vi "script_processor.vi"(7 "Ref_RunScriptWindow":refnum<vi>, 8 "error in (no error)":errorcluster, 10 "command":string) -> (0 "error out":errorcluster)   [LabVIEW 2017]
doc: "This is the main VI that processes all the script command. Here are all the functions listed and processed"
uses:
  Classes/Flags/flag.lvclass
  Classes/Plots/Plots.lvclass
  global variables.vi
  Classes/StatusLog/StatusLog.lvclass
  Classes/Message/Message.lvclass
  Classes/PrepLineObject/PrepLineObject.lvclass
  Classes/Standard/Standard.lvclass
  Classes/Pipette/Pipette.lvclass
  Classes/Instrument/instrument.lvclass
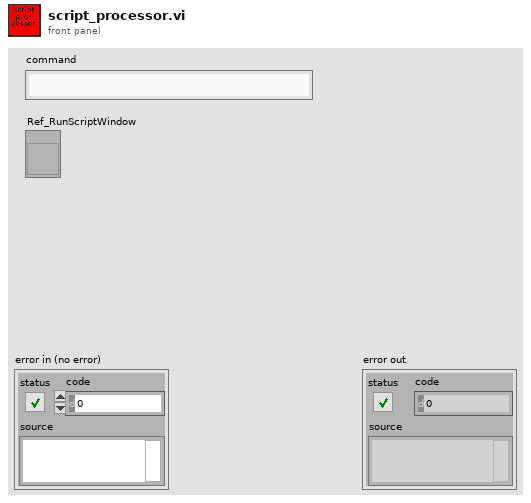
[diagram p1: front panel]
types:
  T1 = cluster{"plot command":string, "Variant":variant}
  T2 = cluster{"format string":string, "Variant":variant}
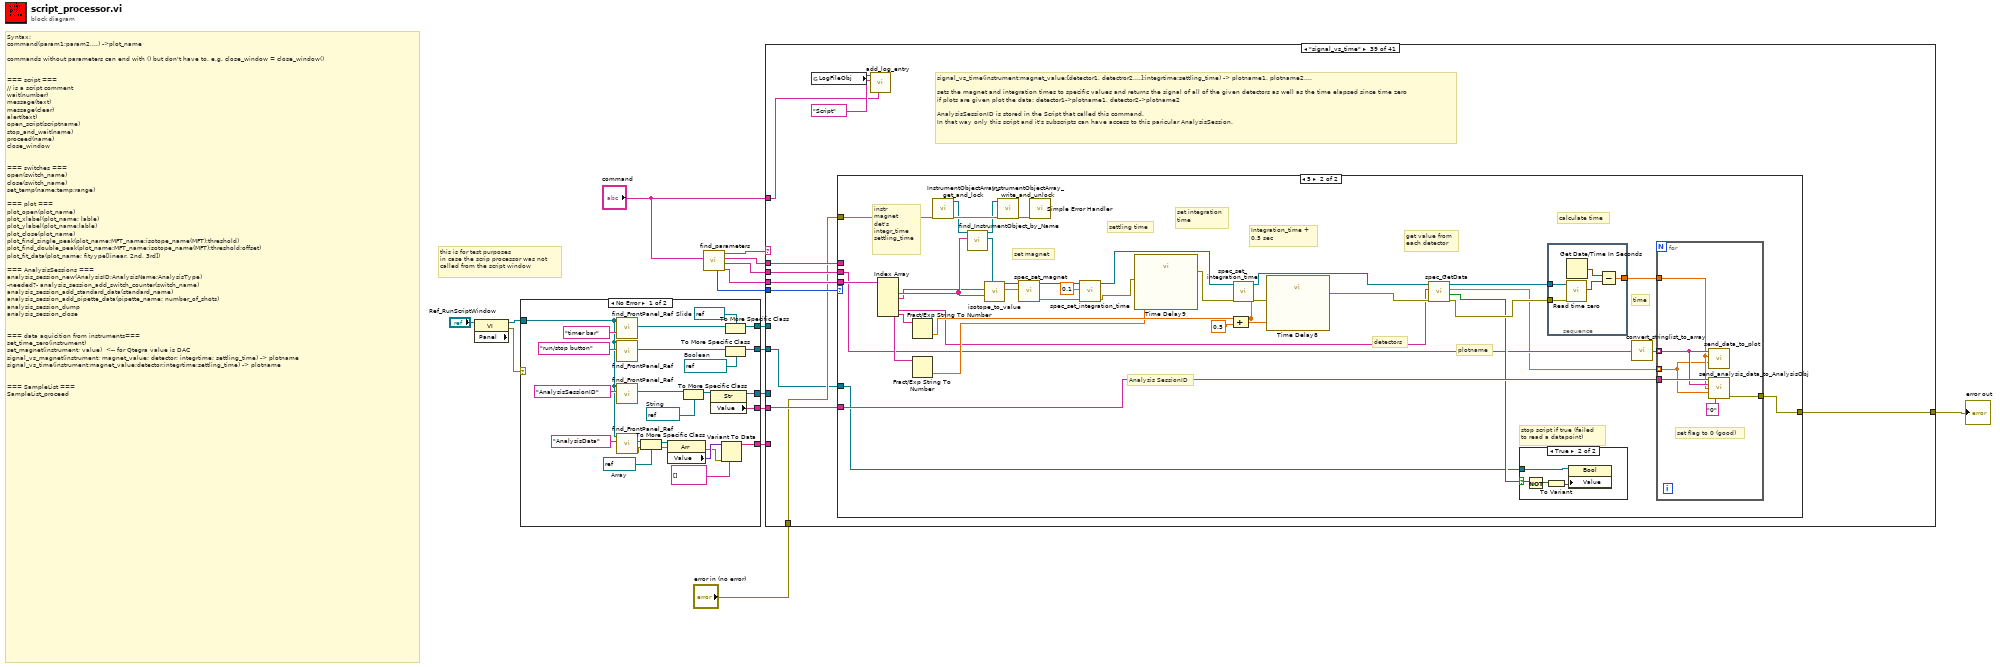
[diagram p0: block diagram]
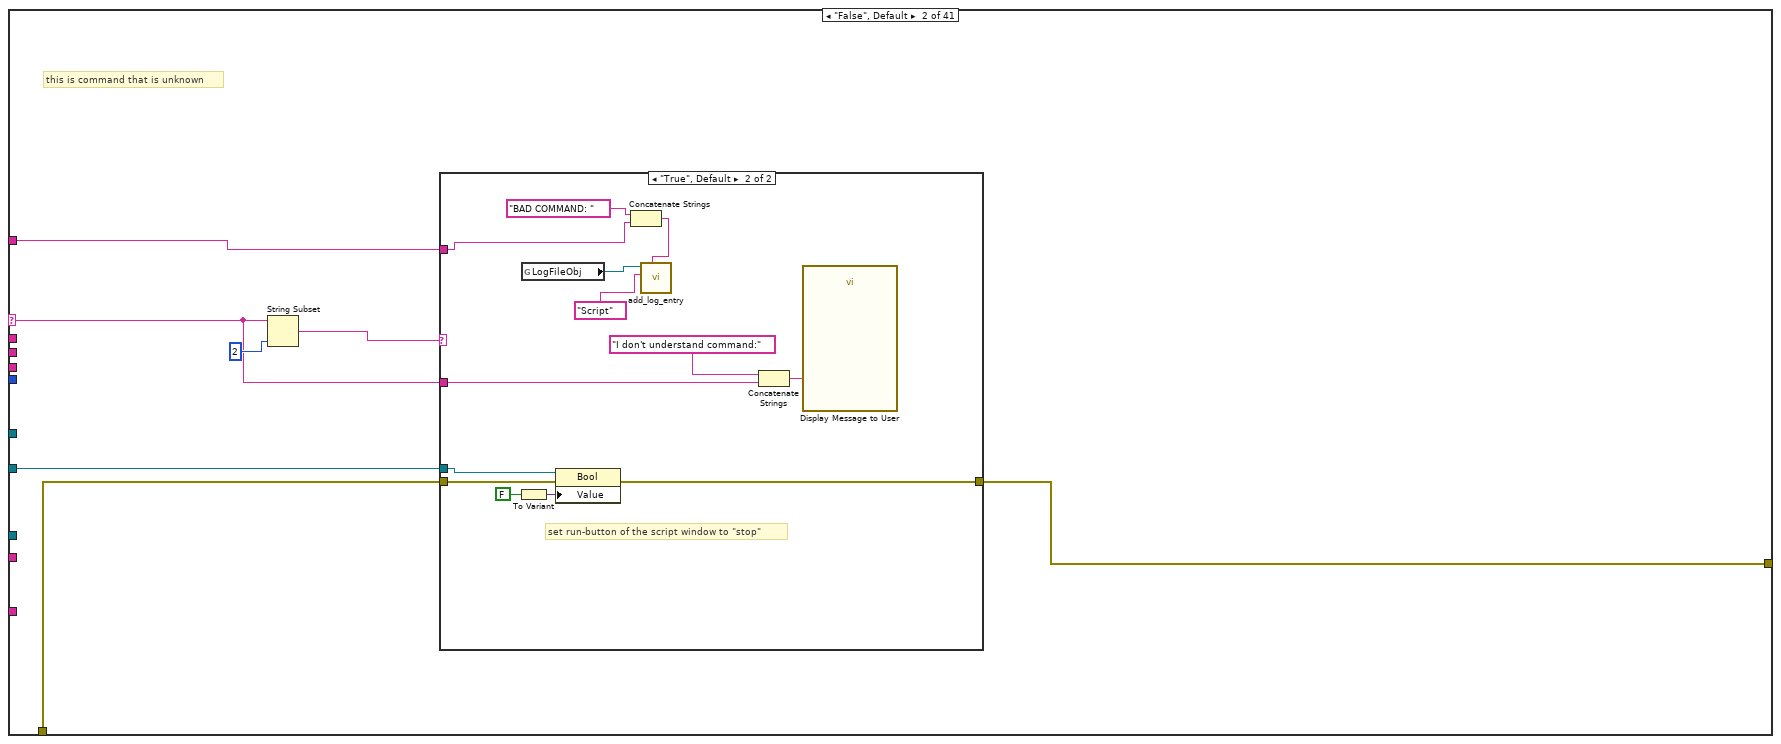
[diagram p4: hidden frame]
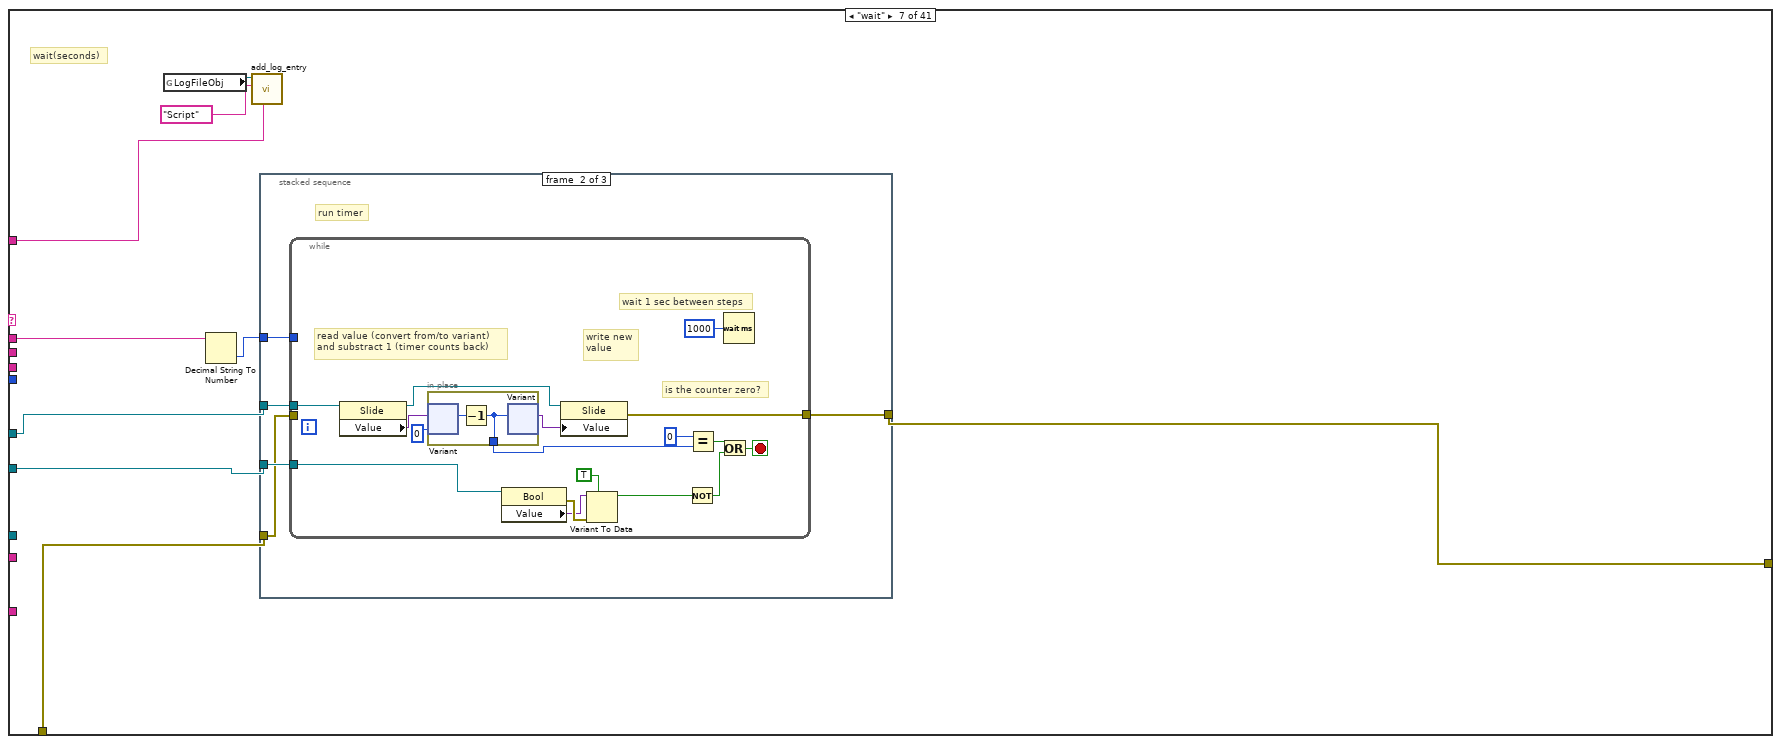
[diagram p10: hidden frame]
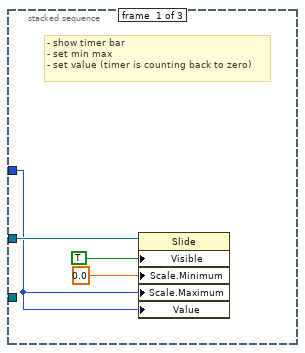
[diagram p11: hidden frame]
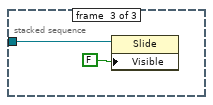
[diagram p12: hidden frame]
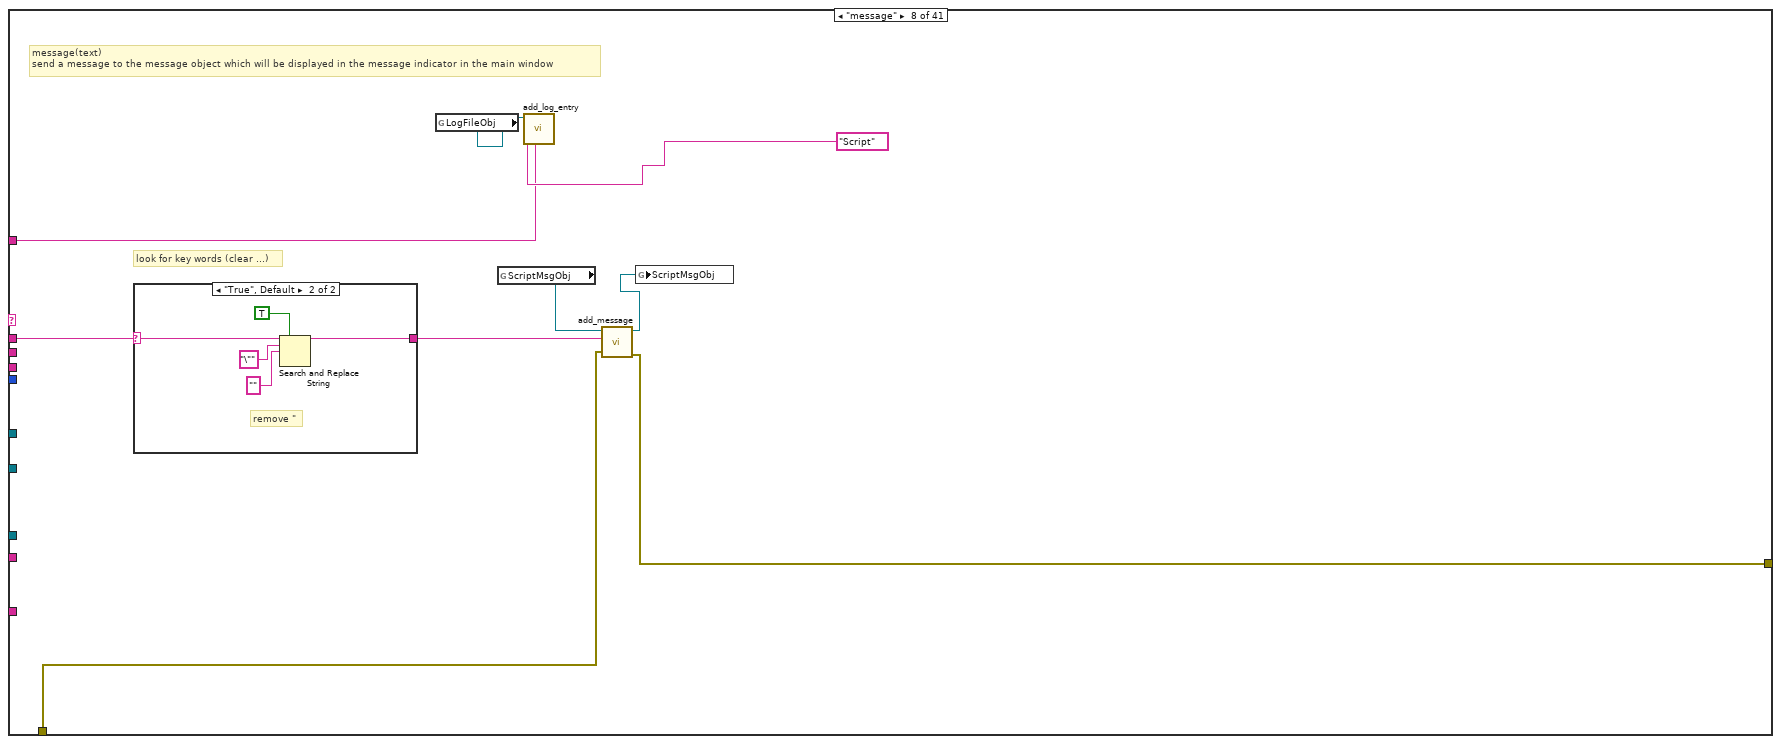
[diagram p13: hidden frame]
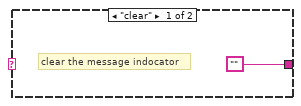
[diagram p14: hidden frame]
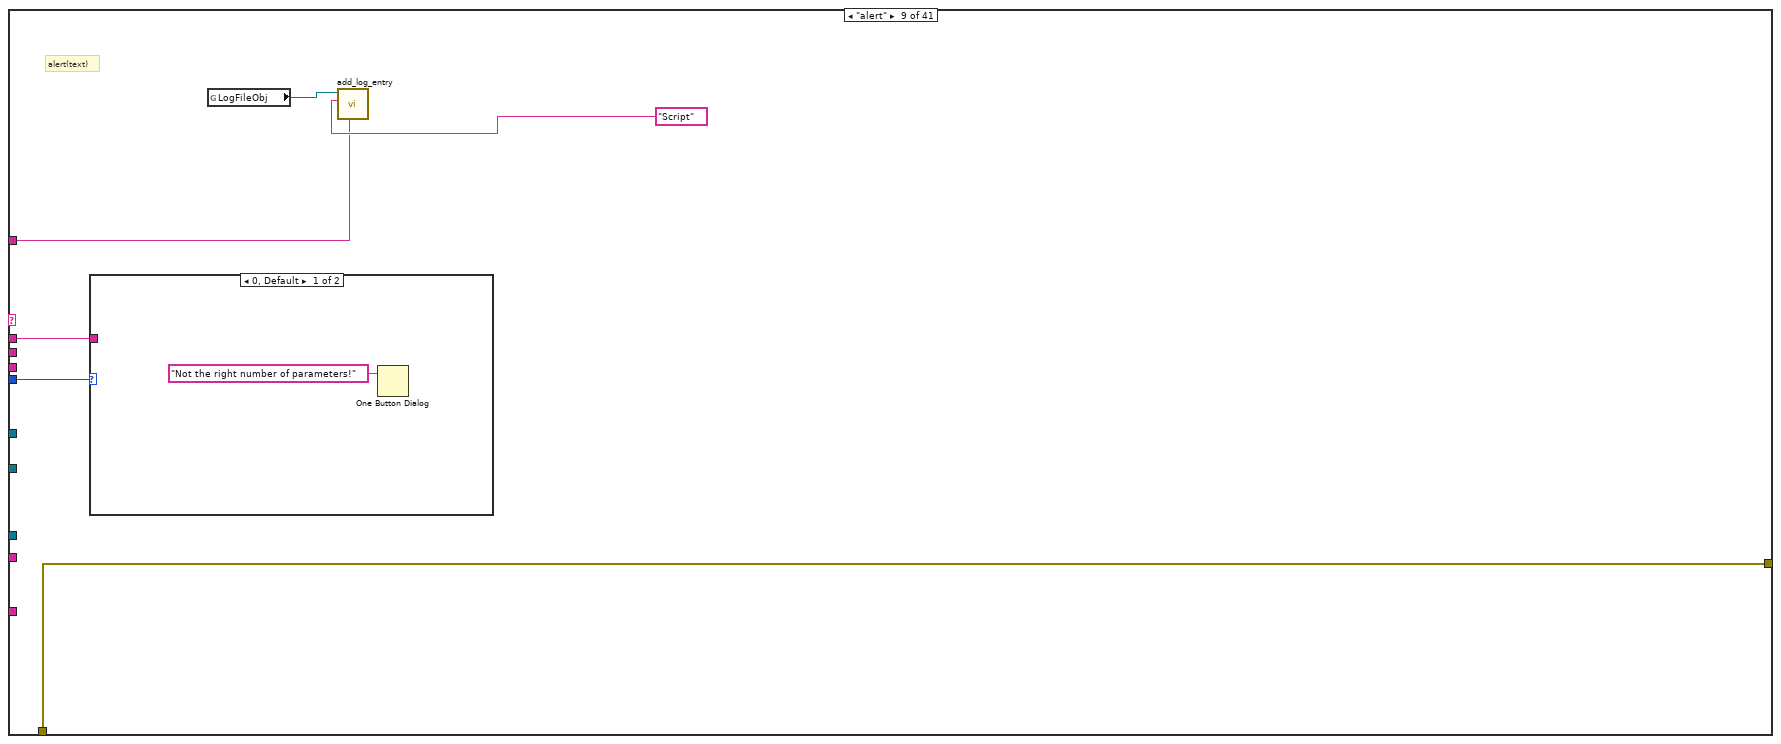
[diagram p15: hidden frame]
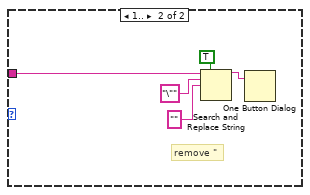
[diagram p16: hidden frame]
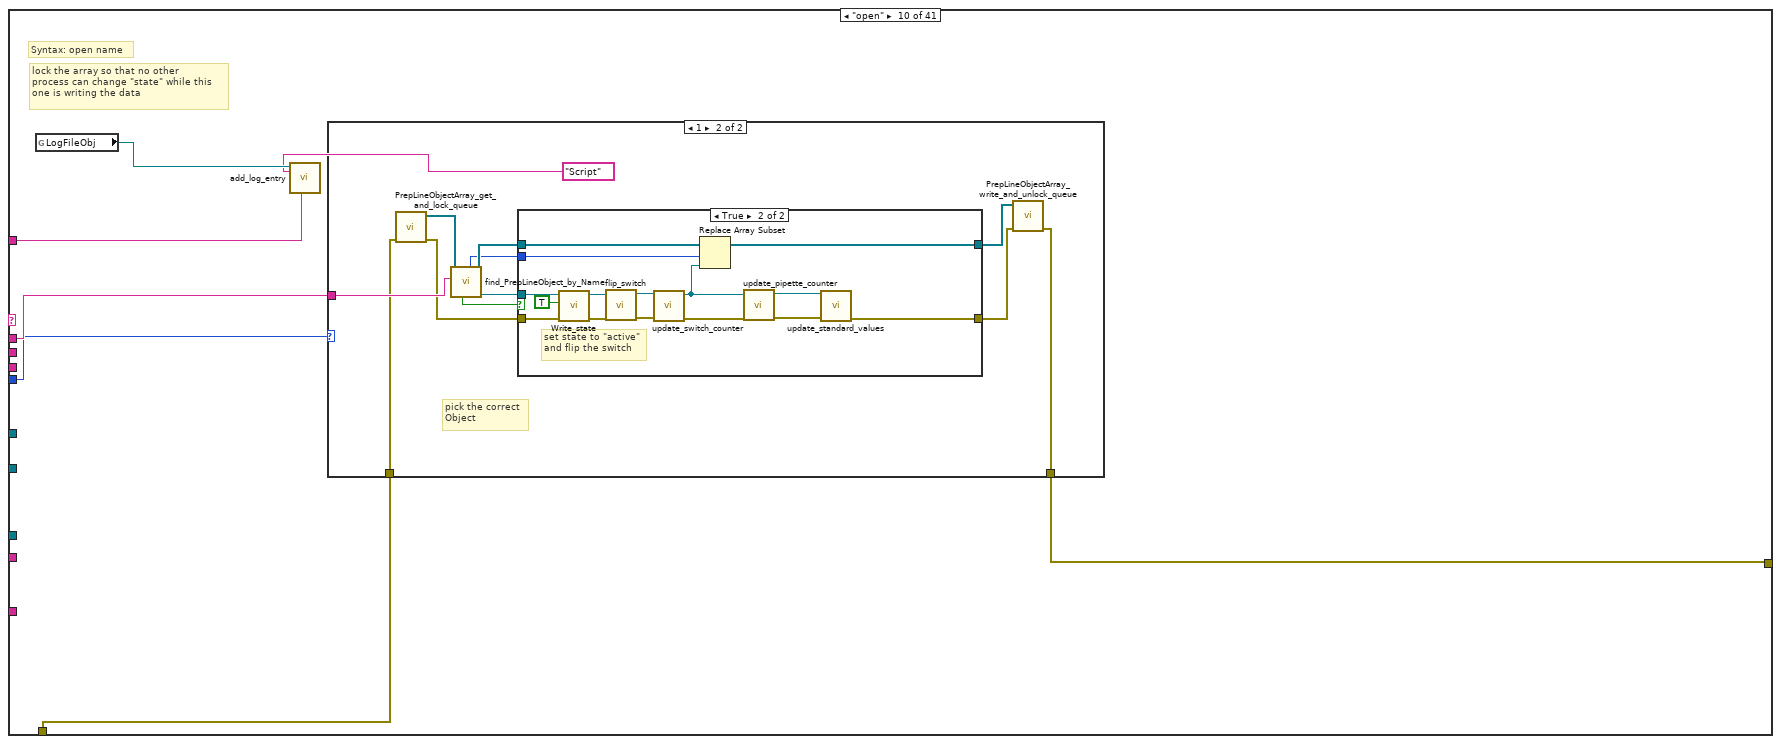
[diagram p17: hidden frame]
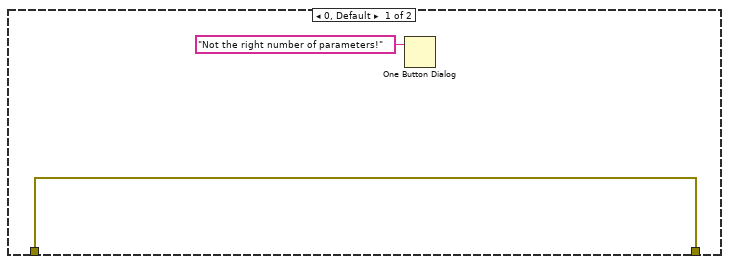
[diagram p18: hidden frame]
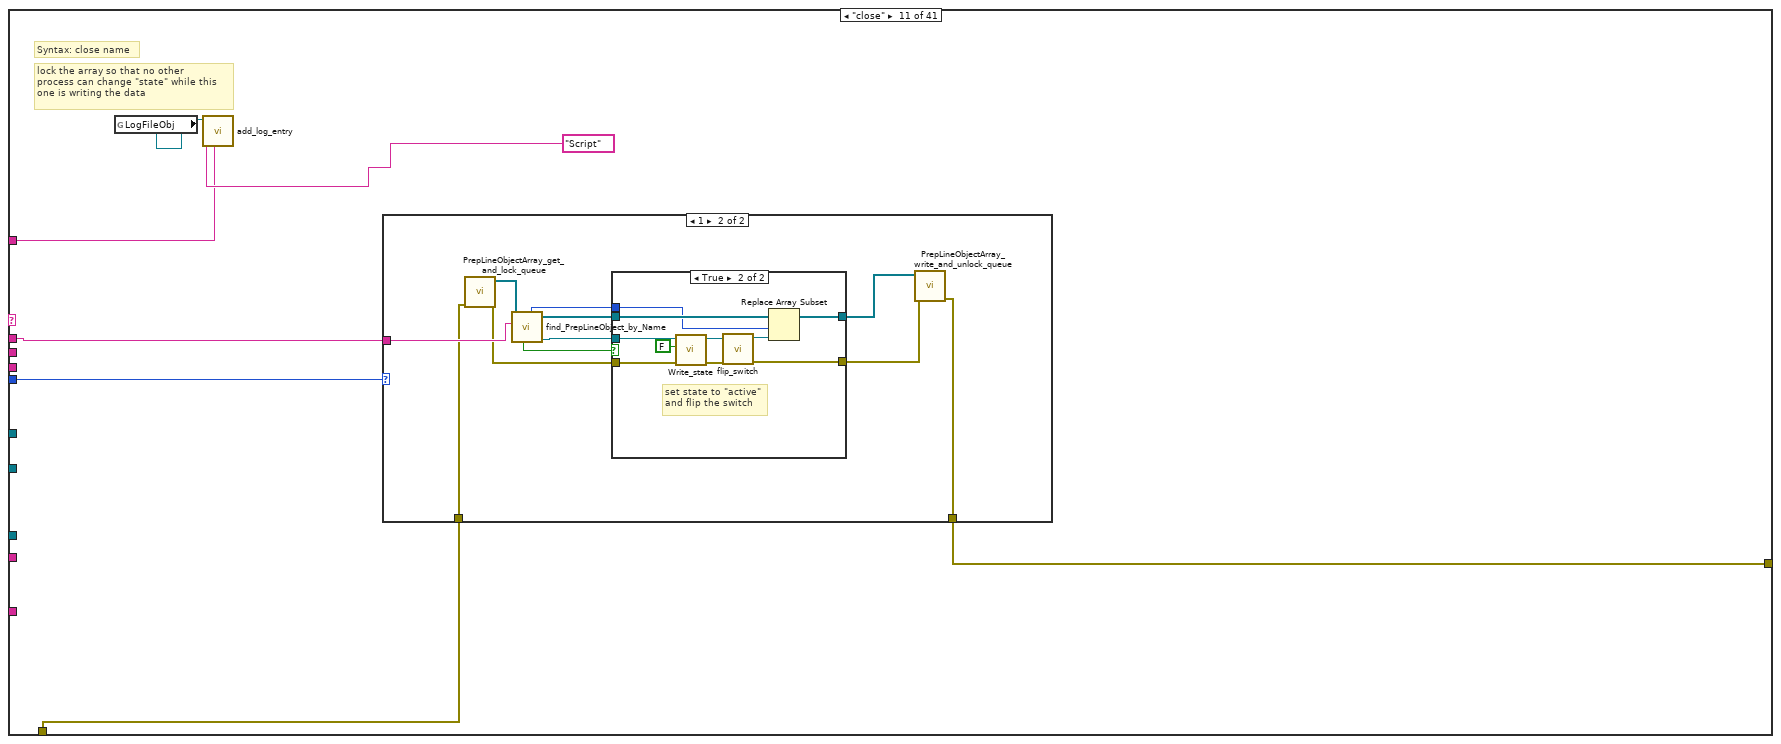
[diagram p20: hidden frame]
diagram:
  # "this is for test purposes\nin case the scrip processor was not\ncalled from the script window"
  # "Syntax:\ncommand(param1;param2,...) ->plot_name\n\ncommands without parameters can end with () but don't have to, e.g. close_window = close_window()\n\n\n=== script ===\n// is a script comment\nwait(number)\nmessage(text)\nmessage(clear)\nalert(text)\nopen_script(scriptname)\nstop_and_wait(name)\nproceed(name)\nclose_window\n\n\n=== switches ===\nopen(switch_name)\nclose(switch_name)\nset_temp(name;temp;range)\n\n=== plot ===\nplot_open(plot_name)\nplot_xlabel(plot_name; lable)\nplot_ylabel(plot_name;lable)\nplot_close(plot_name)\nplot_find_single_peak(plot_name;MFT_name;isotope_name(MFT);threshold)\nplot_find_double_peak(plot_name;MFT_name;isotope_name(MFT);threshold;offset)\nplot_fit_data(plot_name; fityype[linear, 2nd, 3rd])\n\n=== AnalysisSessions ===\nanalysis_session_new(AnalysisID;AnalysisName;AnalysisType)\n-needed?- analysis_session_add_switch_counter(switch_name)\nanalysis_session_add_standard_data(standard_name)\nanalysis_session_add_pipette_data(pipette_name; number_of_shots)\nanalysis_session_dump\nanalysis_session_close\n\n\n=== data aquicition from instruments===\nset_time_zero(instrument)\nset_magnet(instrument; value)  <-- for Qtegra value is DAC\nsignal_vs_magnet(instrument; magnet_value; detector; integrtime; settling_time) -> plotname\nsignal_vs_time(instrument;magnet_value;detector;integrtime;settling_time) -> plotname\n\n\n=== SampleList ===\nSampleList_proceed"
  n1 = property class="VI" props=["Panel"](reference="Ref_RunScriptWindow") -> (reference out=w5:refnum<vi>, error out=w4:errorcluster)  [unwired: 1 in, 1 out]
  n2 = case shown="No Error" w4 {
    tunnel: [w36 _] -> w14
    tunnel: [w35 _] -> w13
    tunnel: w5 -> [w17 _]
    tunnel: [w29 _] -> w3
    tunnel: [w28 _] -> w2
    tunnel: [w22 _] -> w1
    frame No Error {
      w25 = refnum<vi> refnum  # Array
      w32 = refnum<vi> refnum  # String
      w34 = refnum<vi> refnum  # Boolean
      w37 = refnum<vi> refnum  # Slide
      n3 = call "find_FrontPanel_Ref.vi"("FrontPanelObject name"="timer bar", "Ref_RunScriptWindow"=w17) -> ("FrontPanelObject ref out"=w39:refnum<vi>)  [unwired: 7 in, 2 out]
      n4 = call "find_FrontPanel_Ref.vi"("FrontPanelObject name"="run/stop button", "Ref_RunScriptWindow"=w17) -> ("FrontPanelObject ref out"=w38:refnum<vi>)  [unwired: 7 in, 2 out]
      n5 = call "find_FrontPanel_Ref.vi"("FrontPanelObject name"="AnalysisSessionID", "Ref_RunScriptWindow"=w17) -> ("FrontPanelObject ref out"=w31:refnum<vi>)  [unwired: 7 in, 2 out]
      n6 = call "find_FrontPanel_Ref.vi"("FrontPanelObject name"="AnalysisData", "Ref_RunScriptWindow"=w17) -> ("error out"=w20:errorcluster, "FrontPanelObject ref out"=w26:refnum<vi>)  [unwired: 7 in, 1 out]
      n7 = To More Specific Class(target class=w25, reference=w26, error in=w20) -> (specific class reference=w27:refnum<vi>, error out=w19:errorcluster)
      n8 = property class="Arr"(reference=w27, error in=w19) -> (error out=w18:errorcluster, "Value"=w21:variant)  [unwired: 1 out]
      n9 = To More Specific Class(target class=w32, reference=w31) -> (specific class reference=w30:refnum<vi>)  [unwired: 1 in, 1 out]
      n10 = property class="Str"(reference=w30) -> (reference out=w28:refnum<vi>, "Value"=w29:string)  [unwired: 1 in, 1 out]
      n11 = Variant To Data(error in=w18, type=string[] [], Variant=w21) -> (data=w22:string[])  [unwired: 1 out]
      n12 = To More Specific Class(target class=w37, reference=w39) -> (specific class reference=w36:refnum<vi>)  [unwired: 1 in, 1 out]
      n13 = To More Specific Class(target class=w34, reference=w38) -> (specific class reference=w35:refnum<vi>)  [unwired: 1 in, 1 out]
    }
    frame Error {
    }
  }
  n14 = call "find_parameters.vi"("script input"="command") -> ("Parameter Array"=w8:string[], "plotnames (string list)"=w9:string, "parameter string"=w10:string, "command"=w11:string, "number of parameters"=w7:u8)  [unwired: 6 in]
  n15 = case shown="\"signal_vs_time\"" w11 {
    selector: w11 -> [_ w47 _ _ _ _ _ _ _ _ _ _ _ _ _ _ _ _ _ _ _ _ _ _ _ _ _ _ _ _ _ _ _ _ _ _ _ _ _ _ _]
    tunnel: w10 -> [_ _ _ _ _ _ w76 w110 w127 w140 w177 w211 w270 w298 w353 _ w403 w437 w453 w463 w498 w557 w623 _ _ w718 w747 w776 _ w820 w857 w886 w917 w948 w989 w1022 w1053 w1103 w1164 w1227 _]
    tunnel: w13 -> [_ w46 _ _ _ _ w73 _ _ _ _ w210 w261 w297 _ _ _ _ _ _ _ _ _ _ _ _ _ _ _ _ _ _ _ _ _ _ w1046 w1096 w1157 _ _]
    tunnel: "error in (no error)" -> [w42 w45 w64 w65 w66 w67 w72 w113 w122 w139 w176 w209 w269 w291 w352 w390 w410 w436 w452 w468 w499 w558 w624 w683 w712 w715 w744 w773 _ w819 w853 w882 w913 w944 w985 w1018 w1047 w1097 w1158 w1224 w1261]
    tunnel: [w42 w44 w64 w65 w66 w67 w71 w112 w122 w138 w175 w208 w268 w296 w351 w389 w409 w435 w451 w467 w497 w556 w622 w682 w711 w719 w748 w777 _ w818 w852 w881 w912 w943 w984 w1017 w1052 w1101 w1162 _ w1260] -> w15
    tunnel: "command" -> [_ w43 _ _ _ _ w68 w107 w124 w135 w172 w205 w265 w293 w349 w386 w406 w432 w448 w464 w500 w559 w625 w686 w707 w720 w749 w778 w806 w821 w855 w884 w915 w946 w987 w1020 w1054 w1104 w1165 w1229 w1257]
    tunnel: w14 -> [_ _ _ _ _ _ w74 _ _ _ _ _ _ _ _ _ _ _ _ _ _ _ _ _ _ _ _ _ _ _ _ _ _ _ _ _ _ _ _ _ _]
    tunnel: w9 -> [_ _ _ _ _ _ _ _ _ _ _ _ _ _ _ _ _ _ _ _ _ _ _ _ _ _ _ _ _ _ _ _ _ _ _ _ w1051 w1102 w1163 w1226 _]
    tunnel: w8 -> [_ _ _ _ _ _ _ _ _ _ _ w203 _ _ _ _ w404 w430 w446 _ w495 w554 w620 w677 _ _ _ _ _ _ w851 w880 w911 w942 w983 w1016 w1049 w1099 w1160 w1225 _]
    tunnel: w7 -> [_ _ _ _ _ _ _ _ w123 w134 w171 w204 w264 w292 w348 _ w405 w431 w447 w462 w496 w555 w621 _ _ w717 w746 w775 _ w817 w854 w883 w914 w945 w986 w1019 w1050 w1100 w1161 w1228 _]
    tunnel: w3 -> [_ _ _ _ _ _ _ _ _ _ _ _ w263 _ _ _ _ _ _ _ w494 w553 w619 _ w705 w716 w745 w774 w809 _ _ _ _ _ _ _ w1048 w1098 w1159 w1223 _]
    tunnel: w2 -> [_ _ _ _ _ _ _ _ _ _ _ _ _ _ _ _ _ _ _ _ _ _ _ w679 _ _ _ _ _ _ _ _ _ _ _ _ _ _ _ _ _]
    tunnel: w1 -> [_ _ _ _ _ _ _ _ _ _ _ _ _ _ _ _ _ _ _ _ _ _ _ w675 _ _ _ _ _ _ _ _ _ _ _ _ _ _ _ _ _]
    frame "" {
      # "empty line"
    }
    frame "False", Default {
      # "this is command that is unknown"
      n16 = String Subset(string=w47, length (rest)=2 ("length (rest)")) -> (substring=w48:string)  [unwired: 1 in]
      n17 = case shown="\"True\", Default" w48 {
        tunnel: w47 -> [_ w61]
        tunnel: w46 -> [_ w57]
        tunnel: w45 -> [w50 w58]
        tunnel: [w50 w56] -> w44
        tunnel: w43 -> [_ w51]
        frame "//" {
          # "this is a comment that has no space after it"
        }
        frame "True", Default {
          # "set run-button of the script window to \"stop\""
          n18 = To Variant(anything=FALSE) -> (Variant=w60:variant)
          n19 = global read "global variables.vi" "LogFileObj"() -> (w52:refnum<class "StatusLog.lvclass">)
          n20 = property class="Bool"(reference=w57, error in=w58, "Value"=w60) -> (error out=w56:errorcluster)  [unwired: 1 out]
          n21 = Concatenate Strings("BAD COMMAND: ", w51) -> (w55:string)
          n22 = call-dynamic "add_log_entry.vi"("new entry"=w55, "log identifiers"="Script", "StatusLog in"=w52) -> ()  [unwired: 5 in, 2 out]
          n23 = Concatenate Strings("I don't understand command:" ("Message"), w61) -> (w62:string)
          n24 = call "Display Message to User"("Message"=w62) -> ()  [unwired: 9 in, 2 out]
        }
      }
    }
    frame "\n" {
      # "empty line"
    }
    frame "\r" {
    }
    frame "\n\r" {
    }
    frame "//" {
      # "this is a script comment"
    }
    frame "wait" {
      # "wait(seconds)"
      n25 = global read "global variables.vi" "LogFileObj"() -> (w70:refnum<class "StatusLog.lvclass">)
      n26 = Decimal String To Number(string=w76) -> (number=w75:i32)  [unwired: 2 in, 1 out]
      n27 = call-dynamic "add_log_entry.vi"("new entry"=w68, "log identifiers"="Script", "StatusLog in"=w70) -> ()  [unwired: 5 in, 2 out]
      n28 = stacked-sequence {
        tunnel: w75 -> [w77 w83 _]
        tunnel: w74 -> [w78 w85 w106]
        tunnel: w73 -> [_ w84 _]
        tunnel: w72 -> [_ w82 _]
        tunnel: [_ w81 _] -> w71
        frame #0 {
          # "- show timer bar\n- set min max\n- set value (timer is counting back to zero)"
          n29 = property class="Slide"(reference=w78, "Visible"=TRUE, "Scale.Minimum"=0.0 ("Scale.Range:Minimum"), "Scale.Maximum"=w77, "Value"=w77) -> ()  [unwired: 1 in, 2 out]
        }
        frame #1 {
          # "run timer"
          n30 = while {
            tunnel: w85 -> [w92]
            tunnel: w84 -> [w98]
            tunnel: w83 -> [_]
            tunnel: w82 -> [_]
            tunnel: [w93] -> w81
            stop <- w99 stop-if-true
            # "is the counter zero?"
            # "write new\nvalue"
            # "read value (convert from/to variant)\nand substract 1 (timer counts back)"
            # "wait 1 sec between steps"
            n31 = property class="Slide"(reference=w92) -> (reference out=w86:refnum<vi>, "Value"=w91:variant)  [unwired: 1 in, 1 out]
            n32 = in-place {
              in-place-border: [w103] -> w88
              n33 = in-place-variant #1(w91, u32 0) -> (w104:u32)  [unwired: 1 out]
              n34 = Decrement(x=w104) -> (x-1=w103:u32)
              n35 = in-place-variant #1(w103) -> (w89:variant)  [unwired: 1 out]
            }
            n36 = property class="Bool"(reference=w98) -> (error out=w97:errorcluster, "Value"=w96:variant)  [unwired: 1 in, 1 out]
            n37 = property class="Slide"(reference=w86, "Value"=w89) -> (error out=w93:errorcluster)  [unwired: 1 in, 1 out]
            n38 = Variant To Data(error in=w97, type=TRUE, Variant=w96) -> (data=w95:bool)  [unwired: 1 out]
            n39 = Not(x=w95) -> (.not. x?=w100:bool)
            n40 = Equal?(x=u32 0, y=w88) -> (x = y?=w101:bool)
            n41 = Or(x=w101, y=w100) -> (x .or. y?=w99:bool)
            n42 = Wait (ms)(milliseconds to wait=u32 1000) -> ()  [unwired: 1 out]
          }
        }
        frame #2 {
          n43 = property class="Slide"(reference=w106, "Visible"=FALSE) -> ()  [unwired: 1 in, 2 out]
        }
      }
    }
    frame "message" {
      # "look for key words (clear ...)"
      # "message(text)\nsend a message to the message object which will be displayed in the message indicator in the main window"
      n44 = case shown="\"True\", Default" w110 {
        selector: w110 -> [_ w117]
        tunnel: ["" w118] -> w111
        frame "clear" {
          # "clear the message indocator"
        }
        frame "True", Default {
          # "remove \""
          n45 = Search and Replace String(replace all?=TRUE ("replace all? (F)"), input string=w117, search string="\"", replace string="" ("replace string (\"\")")) -> (result string=w118:string)  [unwired: 4 in, 3 out]
        }
      }
      n46 = global read "global variables.vi" "LogFileObj"() -> (w109:refnum<class "StatusLog.lvclass">)
      n47 = global read "global variables.vi" "ScriptMsgObj"() -> (w115:refnum<class "Message.lvclass">)
      n48 = call-dynamic "add_log_entry.vi"("new entry"=w107, "log identifiers"="Script", "StatusLog in"=w109) -> ()  [unwired: 5 in, 2 out]
      n49 = call-dynamic "add_message.vi"("error in (no error)"=w113, "message string"=w111, "Message in"=w115) -> ("error out"=w112:errorcluster, "Message out"=w114:refnum<class "Message.lvclass">)  [unwired: 7 in]
      n50 = global write "global variables.vi" "ScriptMsgObj"(w114) -> ()
    }
    frame "alert" {
      # "alert(text)"
      n51 = case shown="0, Default" w123 {
        tunnel: w127 -> [_ w130]
        frame 0, Default {
          n52 = One Button Dialog(message="Not the right number of parameters!") -> ()  [unwired: 1 in, 1 out]
        }
        frame 1.. {
          # "remove \""
          n53 = Search and Replace String(replace all?=TRUE ("replace all? (F)"), input string=w130, search string="\"", replace string="" ("replace string (\"\")")) -> (result string=w129:string)  [unwired: 4 in, 3 out]
          n54 = One Button Dialog(message=w129) -> ()  [unwired: 1 in, 1 out]
        }
      }
      n55 = global read "global variables.vi" "LogFileObj"() -> (w126:refnum<class "StatusLog.lvclass">)
      n56 = call-dynamic "add_log_entry.vi"("new entry"=w124, "log identifiers"="Script", "StatusLog in"=w126) -> ()  [unwired: 5 in, 2 out]
    }
    frame "open" {
      # "lock the array so that no other\nprocess can change \"state\" while this\none is writing the data"
      # "Syntax: open name"
      n57 = global read "global variables.vi" "LogFileObj"() -> (w137:refnum<class "StatusLog.lvclass">)
      n58 = call-dynamic "add_log_entry.vi"("new entry"=w135, "log identifiers"="Script", "StatusLog in"=w137) -> ()  [unwired: 5 in, 2 out]
      n59 = case shown="1" w134 {
        tunnel: w140 -> [_ w153]
        tunnel: w139 -> [w141 w149]
        tunnel: [w141 w147] -> w138
        frame 0, Default {
          n60 = One Button Dialog(message="Not the right number of parameters!") -> ()  [unwired: 1 in, 1 out]
        }
        frame 1 {
          # "pick the correct\nObject"
          n61 = call "PrepLineObjectArray_get_and_lock_queue.vi"("error in (no error)"=w149) -> ("error out"=w148:errorcluster, "PrepLineObjects"=w151:refnum<class "PrepLineObject.lvclass">[])  [unwired: 9 in]
          n62 = call "find_PrepLineObject_by_Name.vi"("Name of Object"=w153, "PrepLineObjects in"=w151) -> ("found PrepLineObject"=w145:refnum<class "PrepLineObject.lvclass">, "PrepLineObjectsOut"=w152:refnum<class "PrepLineObject.lvclass">[], "index of found"=w146:i32, "found?"=w144:bool)  [unwired: 3 in, 2 out]
          n63 = case shown="True" w144 {
            tunnel: w152 -> [w155 w167]
            tunnel: [w155 w166] -> w150
            tunnel: w148 -> [w154 w165]
            tunnel: w146 -> [_ w162]
            tunnel: w145 -> [_ w161]
            tunnel: [w154 w156] -> w143
            frame False {
            }
            frame True {
              # "set state to \"active\"\nand flip the switch"
              n64 = call-dynamic "Write_state.vi"("error in (no error)"=w165, "state"=TRUE, "PrepLineObject in"=w161) -> ("error out"=w169:errorcluster, "PrepLineObject out"=w170:refnum<class "PrepLineObject.lvclass">)  [unwired: 7 in]
              n65 = call "flip_switch.vi"("PrepLineObject.lvclass"=w170, "error in (no error)"=w169) -> ("PrepLineObject out"=w164:refnum<class "PrepLineObject.lvclass">, "error out"=w163:errorcluster)  [unwired: 7 in]
              n66 = call "update_switch_counter.vi"("PrepLineObject.lvclass"=w164, "error in (no error)"=w163) -> ("PrepLineObject out"=w160:refnum<class "PrepLineObject.lvclass">, "error out"=w159:errorcluster)  [unwired: 7 in]
              n67 = Replace Array Subset(array=w167, new element=w160, index=w162) -> (w166:refnum<class "PrepLineObject.lvclass">[])
              n68 = call "update_pipette_counter.vi"("error in (no error)"=w159, "PrepLineObject in"=w160) -> ("error out"=w157:errorcluster, "PrepLineObject out"=w158:refnum<class "PrepLineObject.lvclass">)  [unwired: 8 in]
              n69 = call "update_standard_values.vi"("error in (no error)"=w157, "PrepLineObject in"=w158) -> ("error out"=w156:errorcluster)  [unwired: 8 in, 1 out]
            }
          }
          n70 = call "PrepLineObjectArray_write_and_unlock_queue.vi"("error in (no error)"=w143, "PrepLineObjArray"=w150) -> ("error out"=w147:errorcluster)  [unwired: 9 in]
        }
      }
    }
    frame "close" {
      # "lock the array so that no other\nprocess can change \"state\" while this\none is writing the data"
      # "Syntax: close name"
      n71 = global read "global variables.vi" "LogFileObj"() -> (w174:refnum<class "StatusLog.lvclass">)
      n72 = call-dynamic "add_log_entry.vi"("new entry"=w172, "log identifiers"="Script", "StatusLog in"=w174) -> ()  [unwired: 5 in, 2 out]
      n73 = case shown="1" w171 {
        tunnel: w177 -> [_ w189]
        tunnel: w176 -> [w178 w186]
        tunnel: [w178 w183] -> w175
        frame 0, Default {
          n74 = One Button Dialog(message="Not the right number of parameters!") -> ()  [unwired: 1 in, 1 out]
        }
        frame 1 {
          n75 = call "PrepLineObjectArray_get_and_lock_queue.vi"("error in (no error)"=w186) -> ("error out"=w185:errorcluster, "PrepLineObjects"=w188:refnum<class "PrepLineObject.lvclass">[])  [unwired: 9 in]
          n76 = call "find_PrepLineObject_by_Name.vi"("Name of Object"=w189, "PrepLineObjects in"=w188) -> ("found PrepLineObject"=w182:refnum<class "PrepLineObject.lvclass">, "PrepLineObjectsOut"=w190:refnum<class "PrepLineObject.lvclass">[], "index of found"=w181:i32, "found?"=w180:bool)  [unwired: 3 in, 2 out]
          n77 = case shown="True" w180 {
            tunnel: w190 -> [w192 w202]
            tunnel: [w192 w198] -> w187
            tunnel: w185 -> [w191 w196]
            tunnel: [w191 w195] -> w184
            tunnel: w182 -> [_ w194]
            tunnel: w181 -> [_ w193]
            frame False {
            }
            frame True {
              # "set state to \"active\"\nand flip the switch"
              n78 = call-dynamic "Write_state.vi"("error in (no error)"=w196, "state"=FALSE, "PrepLineObject in"=w194) -> ("error out"=w200:errorcluster, "PrepLineObject out"=w199:refnum<class "PrepLineObject.lvclass">)  [unwired: 7 in]
              n79 = call "flip_switch.vi"("PrepLineObject.lvclass"=w199, "error in (no error)"=w200) -> ("PrepLineObject out"=w197:refnum<class "PrepLineObject.lvclass">, "error out"=w195:errorcluster)  [unwired: 7 in]
              n80 = Replace Array Subset(array=w202, new element=w197, index=w193) -> (w198:refnum<class "PrepLineObject.lvclass">[])
            }
          }
          n81 = call "PrepLineObjectArray_write_and_unlock_queue.vi"("error in (no error)"=w184, "PrepLineObjArray"=w187) -> ("error out"=w183:errorcluster)  [unwired: 9 in]
        }
      }
    }
    frame "set_temp" {
      # "set_temp(name;temp;range)"
      n82 = global read "global variables.vi" "LogFileObj"() -> (w207:refnum<class "StatusLog.lvclass">)
      n83 = case shown="3" w204 {
        tunnel: w211 -> [_ _]
        tunnel: w210 -> [_ w229]
        tunnel: w209 -> [w212 w226]
        tunnel: [w212 w223] -> w208
        tunnel: w203 -> [_ w219]
        frame 0, Default {
          n84 = One Button Dialog(message="Not the right number of parameters!") -> ()  [unwired: 1 in, 1 out]
        }
        frame 3 {
          # "range"
          # "temp"
          # "- compare value (temp) of the \nPrepLineObject with range\n- when in Range stop the loop"
          # "pick the correct\nObject and set temp"
          n85 = Index Array(array=w219) -> (element #1=w218:string, element #2=w217:string, element #3=w214:string)  [unwired: 3 in]
          n86 = Fract/Exp String To Number(string=w217) -> (number=w216:dbl)  [unwired: 3 in, 1 out]
          n87 = Fract/Exp String To Number(string=w214) -> (number=w215:dbl)  [unwired: 3 in, 1 out]
          n88 = call "PrepLineObjectArray_get_and_lock_queue.vi"("error in (no error)"=w226) -> ("error out"=w225:errorcluster, "PrepLineObjects"=w228:refnum<class "PrepLineObject.lvclass">[])  [unwired: 9 in]
          n89 = call "find_PrepLineObject_by_Name.vi"("Name of Object"=w218, "PrepLineObjects in"=w228) -> ("found PrepLineObject"=w222:refnum<class "PrepLineObject.lvclass">, "PrepLineObjectsOut"=w230:refnum<class "PrepLineObject.lvclass">[], "index of found"=w221:i32, "found?"=w220:bool)  [unwired: 3 in, 2 out]
          n90 = case shown="True" w220 {
            tunnel: w230 -> [w232 w240]
            tunnel: [w232 w239] -> w227
            tunnel: w225 -> [w231 w237]
            tunnel: [w231 w236] -> w224
            tunnel: w216 -> [_ w235]
            tunnel: w222 -> [_ w234]
            tunnel: w221 -> [_ w233]
            frame False {
            }
            frame True {
              n91 = call "set_temperature.vi"("PrepLineObject.lvclass"=w234, "temperature"=w235, "error in (no error)"=w237) -> ("PrepLineObject out"=w238:refnum<class "PrepLineObject.lvclass">, "error out"=w236:errorcluster)  [unwired: 6 in]
              n92 = Replace Array Subset(array=w240, new element=w238, index=w233) -> (w239:refnum<class "PrepLineObject.lvclass">[])
            }
          }
          n93 = call "PrepLineObjectArray_write_and_unlock_queue.vi"("error in (no error)"=w224, "PrepLineObjArray"=w227) -> ("error out"=w223:errorcluster)  [unwired: 9 in]
          n94 = while {
            tunnel: w215 -> [w243]
            tunnel: w229 -> [w258]
            tunnel: w218 -> [w248]
            tunnel: w216 -> [w242]
            stop <- w259 stop-if-true
            n95 = call "PrepLineObjectArray_get_and_lock_queue.vi"() -> ("PrepLineObjects"=w246:refnum<class "PrepLineObject.lvclass">[])  [unwired: 10 in, 1 out]
            n96 = call "find_PrepLineObject_by_Name.vi"("Name of Object"=w248, "PrepLineObjects in"=w246) -> ("found PrepLineObject"=w247:refnum<class "PrepLineObject.lvclass">, "PrepLineObjectsOut"=w245:refnum<class "PrepLineObject.lvclass">[])  [unwired: 3 in, 4 out]
            n97 = call-dynamic "Read_value.vi"("PrepLineObject in"=w247) -> ("error out"=w244:errorcluster, "value"=w255:string)  [unwired: 8 in, 1 out]
            n98 = property class="Bool"(reference=w258) -> (error out=w252:errorcluster, "Value"=w251:variant)  [unwired: 1 in, 1 out]
            n99 = Fract/Exp String To Number(string=w255) -> (number=w241:dbl)  [unwired: 3 in, 1 out]
            n100 = call "PrepLineObjectArray_write_and_unlock_queue.vi"("error in (no error)"=w244, "PrepLineObjArray"=w245) -> ()  [unwired: 9 in, 1 out]
            n101 = Add(x=w243, y=w242) -> (x+y=w254:dbl)
            n102 = Subtract(x=w242, y=w243) -> (x-y=w253:dbl)
            n103 = Variant To Data(error in=w252, type=TRUE, Variant=w251) -> (data=w249:bool)  [unwired: 1 out]
            n104 = In Range and Coerce(upper limit=w254, x=w241, lower limit=w253) -> (In Range?=w260:bool)  [unwired: 1 out]
            n105 = Not(x=w249) -> (.not. x?=w257:bool)
            n106 = Or(x=w260, y=w257) -> (x .or. y?=w259:bool)
            n107 = Wait (ms)(milliseconds to wait=u32 1000) -> ()  [unwired: 1 out]
          }
        }
      }
      n108 = call-dynamic "add_log_entry.vi"("new entry"=w205, "log identifiers"="Script", "StatusLog in"=w207) -> ()  [unwired: 5 in, 2 out]
    }
    frame "open_script" {
      # "open_script(script_name)"
      # "inherit AnalysisSessionID"
      # "opens a new script window with the selected script\nThe script must be in the \"RunScripts\" folder.\n\nThe value of AnalysisSessionID is inherited to the subscript.\nThat way the subscript has access to the same AnalysisSession in order to save data."
      n109 = global read "global variables.vi" "LogFileObj"() -> (w267:refnum<class "StatusLog.lvclass">)
      n110 = global read "global variables.vi" "RunScriptsFolder"() -> (w262:path)
      n111 = call-dynamic "add_log_entry.vi"("new entry"=w265, "log identifiers"="Script", "StatusLog in"=w267) -> ()  [unwired: 5 in, 2 out]
      n112 = case shown="1" w264 {
        tunnel: w270 -> [_ w280]
        tunnel: w269 -> [w272 w279]
        tunnel: [w272 w278] -> w268
        tunnel: w263 -> [_ w277]
        tunnel: w262 -> [_ w276]
        tunnel: w261 -> [_ w273]
        frame 0, Default {
          n113 = One Button Dialog(message="Not the right number of parameters!") -> ()  [unwired: 1 in, 1 out]
        }
        frame 1 {
          # "check if file\nexists"
          n114 = Build Path(base path=w276, name or relative path=w280) -> (appended path=w275:path)
          n115 = Open/Create/Replace File(file path (use dialog)=w275) -> (error out=w274:errorcluster)  [unwired: 5 in, 2 out]
          n116 = case shown="No Error" w274 {
            tunnel: w279 -> [w284 w290]
            tunnel: [w283 w290] -> w278
            tunnel: w277 -> [w282 _]
            tunnel: w275 -> [w281 _]
            tunnel: w273 -> [_ w287]
            frame No Error {
              # "start the script"
              n117 = call "open_Script_Window_dyn.vi"("AnalysisSessionID"=w282, "error in (no error)"=w284, "run/stop button"=TRUE, "Script Path"=w281) -> ("error out"=w283:errorcluster)  [unwired: 7 in]
            }
            frame Error {
              # "stop script"
              n118 = To Variant(anything=FALSE) -> (Variant=w288:variant)
              n119 = property class="Bool"(reference=w287, "Value"=w288) -> ()  [unwired: 1 in, 2 out]
              n120 = One Button Dialog(message="script file doesn't\nexist!!!") -> ()  [unwired: 1 in, 1 out]
            }
          }
        }
      }
    }
    frame "stop_and_wait" {
      # "creates a flag (from the flag array stored in a queue)\nand waits for the flag to be false"
      n121 = global read "global variables.vi" "LogFileObj"() -> (w295:refnum<class "StatusLog.lvclass">)
      n122 = call-dynamic "add_log_entry.vi"("new entry"=w293, "log identifiers"="Script", "StatusLog in"=w295) -> ()  [unwired: 5 in, 2 out]
      n123 = case shown="1" w292 {
        tunnel: w298 -> [_ w304]
        tunnel: w297 -> [_ w303]
        tunnel: w291 -> [w299 w302]
        tunnel: [w299 w301] -> w296
        frame 0, Default {
          n124 = One Button Dialog(message="Not the right number of parameters!") -> ()  [unwired: 1 in, 1 out]
        }
        frame 1 {
          n125 = while {
            tunnel: w304 -> [w316]
            tunnel: w303 -> [w313]
            tunnel: w302 -> [w308]
            tunnel: [w305] -> w301
            stop <- w315 continue-if-true
            # "run until flag is false"
            n126 = call "FlagObjectArray_get_and_lock.vi"("error in (no error)"=w308) -> ("error out"=w307:errorcluster, "FlagObjects"=w311:refnum<class "flag.lvclass">[])  [unwired: 9 in]
            n127 = call "find_FlagObject_by_Name.vi"("Flag Name"=w316, "FlagObj Array"=w311) -> ("index of Object in Array"=w309:i32, "found?"=w318:bool, "found FlagObj out"=w314:refnum<class "flag.lvclass">, "FlagObj Array out"=w317:refnum<class "flag.lvclass">[])  [unwired: 6 in]
            n128 = case shown="True" w318 {
              tunnel: w317 -> [w328 w335]
              tunnel: w316 -> [w329 _]
              tunnel: [TRUE w336] -> w315
              tunnel: w314 -> [_ w342]
              tunnel: w313 -> [_ w341]
              tunnel: [w321 w332] -> w310
              tunnel: w309 -> [_ w333]
              tunnel: w307 -> [w320 w331]
              tunnel: [w319 w330] -> w306
              frame False {
                # "flag does not exist -> create\nand set to true"
                n129 = call-dynamic "Write_flag-name.vi"("error in (no error)"=w320, "flag name"=w329, "flag in"=refnum<class "flag.lvclass"> refnum ("flag.lvclass")) -> ("error out"=w325:errorcluster, "flag out"=w326:refnum<class "flag.lvclass">)  [unwired: 7 in]
                n130 = call-dynamic "Write_flag-state.vi"("error in (no error)"=w325, "flag state"=TRUE, "flag in"=w326) -> ("error out"=w319:errorcluster, "flag out"=w323:refnum<class "flag.lvclass">)  [unwired: 7 in]
                n131 = Build Array (concatenate)(w328, w323) -> (w321:refnum<class "flag.lvclass">[])
              }
              frame True {
                # "flag exists already. check if flag is false\n(\"proceed\" happened), then destroy the flag"
                n132 = property class="Bool"(reference=w341) -> (error out=w340:errorcluster, "Value"=w339:variant)  [unwired: 1 in, 1 out]
                n133 = call-dynamic "Read_flag-state.vi"("error in (no error)"=w331, "flag in"=w342) -> ("error out"=w330:errorcluster, "flag state"=w334:bool)  [unwired: 7 in, 1 out]
                n134 = Variant To Data(error in=w340, type=FALSE, Variant=w339) -> (data=w337:bool)  [unwired: 1 out]
                n135 = And(x=w334, y=w337) -> (x .and. y?=w336:bool)
                n136 = case shown="False" w334 {
                  tunnel: w335 -> [w345 w346]
                  tunnel: w333 -> [w344 _]
                  tunnel: [w343 w346] -> w332
                  frame False {
                    n137 = Delete From Array(array=w345, index=w344) -> (array with subset deleted=w343:refnum<class "flag.lvclass">[])  [unwired: 1 in, 1 out]
                  }
                  frame True {
                  }
                }
              }
            }
            n138 = call "FlagObjectArray_write_and_unlock.vi"("error in (no error)"=w306, "FlagObjects"=w310) -> ("error out"=w305:errorcluster)  [unwired: 9 in]
            n139 = Wait (ms)(milliseconds to wait=u32 500) -> ()  [unwired: 1 out]
          }
        }
      }
    }
    frame "proceed" {
      # "creates a flag (from the flag array stored in a queue)\nand waits for the flag to be false"
      n140 = global read "global variables.vi" "LogFileObj"() -> (w350:refnum<class "StatusLog.lvclass">)
      n141 = call-dynamic "add_log_entry.vi"("new entry"=w349, "log identifiers"="Script", "StatusLog in"=w350) -> ()  [unwired: 5 in, 2 out]
      n142 = case shown="1" w348 {
        tunnel: w353 -> [_ w366]
        tunnel: w352 -> [w354 w359]
        tunnel: [w354 w356] -> w351
        frame 0, Default {
          n143 = One Button Dialog(message="Not the right number of parameters!") -> ()  [unwired: 1 in, 1 out]
        }
        frame 1 {
          n144 = call "FlagObjectArray_get_and_lock.vi"("error in (no error)"=w359) -> ("error out"=w358:errorcluster, "FlagObjects"=w361:refnum<class "flag.lvclass">[])  [unwired: 9 in]
          n145 = call "find_FlagObject_by_Name.vi"("Flag Name"=w366, "FlagObj Array"=w361) -> ("index of Object in Array"=w362:i32, "found?"=w365:bool, "found FlagObj out"=w363:refnum<class "flag.lvclass">, "FlagObj Array out"=w364:refnum<class "flag.lvclass">[])  [unwired: 6 in]
          n146 = case shown="True" w365 {
            tunnel: w364 -> [w375 w382]
            tunnel: w366 -> [w376 _]
            tunnel: w363 -> [_ w384]
            tunnel: [w369 w379] -> w360
            tunnel: w362 -> [_ w380]
            tunnel: w358 -> [w368 w378]
            tunnel: [w367 w377] -> w357
            frame False {
              # "flag does not exist which means that\nstop_and_wait hasn't happened yet\n-> create and set to false"
              n147 = call-dynamic "Write_flag-name.vi"("error in (no error)"=w368, "flag name"=w376, "flag in"=refnum<class "flag.lvclass"> refnum ("flag.lvclass")) -> ("error out"=w372:errorcluster, "flag out"=w373:refnum<class "flag.lvclass">)  [unwired: 7 in]
              n148 = call-dynamic "Write_flag-state.vi"("error in (no error)"=w372, "flag state"=FALSE, "flag in"=w373) -> ("error out"=w367:errorcluster, "flag out"=w370:refnum<class "flag.lvclass">)  [unwired: 7 in]
              n149 = Build Array (concatenate)(w375, w370) -> (w369:refnum<class "flag.lvclass">[])
            }
            frame True {
              # "flag exists already which means that\na \"stop_and_wait\" is waiting somewhere\n->set to false"
              n150 = call-dynamic "Write_flag-state.vi"("error in (no error)"=w378, "flag state"=FALSE, "flag in"=w384) -> ("error out"=w377:errorcluster, "flag out"=w381:refnum<class "flag.lvclass">)  [unwired: 7 in]
              n151 = Replace Array Subset(array=w382, new element=w381, index=w380) -> (w379:refnum<class "flag.lvclass">[])
              n152 = Wait (ms)(milliseconds to wait=u32 250) -> ()  [unwired: 1 out]
            }
          }
          n153 = call "FlagObjectArray_write_and_unlock.vi"("error in (no error)"=w357, "FlagObjects"=w360) -> ("error out"=w356:errorcluster)  [unwired: 9 in]
        }
      }
    }
    frame "close_window" {
      # "find the VI that has called\nthe command"
      # "close window"
      # "set button to false"
      # "closes the script window of the the VI that calls the command"
      n154 = global read "global variables.vi" "LogFileObj"() -> (w388:refnum<class "StatusLog.lvclass">)
      n155 = call-dynamic "add_log_entry.vi"("new entry"=w386, "log identifiers"="Script", "StatusLog in"=w388) -> ()  [unwired: 5 in, 2 out]
      n156 = Call Chain() -> (call chain=w402:string[])
      n157 = Array Size(array=w402) -> (size(s)=w401:i32)
      n158 = Decrement(x=w401) -> (x-1=w397:i32)
      n159 = Index Array(array=w402, index=w397) -> (element=w392:string)
      n160 = Open VI Reference(vi path=w392, error in (no error)=w390) -> (vi reference=w400:refnum<vi>, error out=w399:errorcluster)  [unwired: 4 in]
      n161 = invoke class="VI" method="Ctrl Val.Set"(reference=w400, error in=w399, "Control Name"="run/stop button", "Value"=FALSE) -> (reference out=w394:refnum<vi>, error out=w393:errorcluster)  [unwired: 1 in, 3 out]
      n162 = invoke class="VI" method="FP.Close"(reference=w394, error in=w393) -> (reference out=w395:refnum<vi>, error out=w396:errorcluster)  [unwired: 1 in, 1 out]
      n163 = Close Reference(reference=w395, error in (no error)=w396) -> (error out=w389:errorcluster)
    }
    frame "plot_open" {
      n164 = global read "global variables.vi" "LogFileObj"() -> (w408:refnum<class "StatusLog.lvclass">)
      n165 = call-dynamic "add_log_entry.vi"("new entry"=w406, "log identifiers"="Script", "StatusLog in"=w408) -> ()  [unwired: 5 in, 2 out]
      n166 = case shown="1" w405 {
        tunnel: w410 -> [w411 w426]
        tunnel: [w411 w419] -> w409
        tunnel: w404 -> [_ _]
        tunnel: w403 -> [_ w413]
        frame 0, Default {
          n167 = One Button Dialog(message="Not the right number of parameters!") -> ()  [unwired: 1 in, 1 out]
        }
        frame 1 {
          # "plotname=isotopename"
          # "IsotopeName"
          # "plotname"
          # "instantiates a plot object\nopens a plot window \nwrite new plot object to global queue"
          n168 = call "PlotObjectArray_get_and_lock.vi"("error in (no error)"=w426) -> ("error out"=w425:errorcluster, "PlotObjects"=w428:refnum<class "Plots.lvclass">[])  [unwired: 9 in]
          n169 = call-dynamic "Write_PlotID.vi"("error in (no error)"=w425, "PlotID"=w413, "Plots in"=refnum<class "Plots.lvclass"> refnum ("Plots.lvclass")) -> ("error out"=w422:errorcluster, "Plots out"=w423:refnum<class "Plots.lvclass">)  [unwired: 7 in]
          n170 = Concatenate Strings("plot_cmd_" ("string"), w413) -> (w421:string)
          n171 = call-dynamic "Write cmd queue name.vi"("error in (no error)"=w422, "cmd queue name"=w421, "Plots in"=w423) -> ("error out"=w416:errorcluster, "Plots out"=w417:refnum<class "Plots.lvclass">)  [unwired: 7 in]
          n172 = call-dynamic "Write IsotopeID.vi"("error in (no error)"=w416, "IsotopeID"=w413, "Plots in"=w417) -> ("error out"=w414:errorcluster, "Plots out"=w415:refnum<class "Plots.lvclass">)  [unwired: 7 in]
          n173 = Build Array (concatenate)(w428, w415) -> (w427:refnum<class "Plots.lvclass">[])
          n174 = call "PlotObjectArray_write_and_unlock.vi"("error in (no error)"=w414, "PlotObjects"=w427) -> ("error out"=w420:errorcluster)  [unwired: 9 in]
          n175 = Wait (ms)(milliseconds to wait=u32 500) -> ()  [unwired: 1 out]
          n176 = call "load_plot_window_dyn_2.vi"("error in (no error)"=w420, "Plots in"=w415) -> ("error out"=w419:errorcluster)  [unwired: 8 in, 1 out]
        }
      }
    }
    frame "plot_xlabel" {
      # "writes the private property \"xlabel\" to the plot object with the correct plotID"
      n177 = case shown="2" w431 {
        tunnel: w437 -> [_ _]
        tunnel: w436 -> [w438 w445]
        tunnel: [w438 w444] -> w435
        tunnel: w430 -> [_ w443]
        frame 0, Default {
          n178 = One Button Dialog(message="Not the right number of parameters!") -> ()  [unwired: 1 in, 1 out]
        }
        frame 2 {
          n179 = Index Array(array=w443) -> (element #1=w442:string, element #2=w441:string)  [unwired: 2 in]
          n180 = call "plot_set_labels.vi"("error in (no error)"=w445, "label"=w441, "axis"="xlabel", "plot name"=w442) -> ("error out"=w444:errorcluster)  [unwired: 7 in]
        }
      }
      n181 = global read "global variables.vi" "LogFileObj"() -> (w434:refnum<class "StatusLog.lvclass">)
      n182 = call-dynamic "add_log_entry.vi"("new entry"=w432, "log identifiers"="Script", "StatusLog in"=w434) -> ()  [unwired: 5 in, 2 out]
    }
    frame "plot_ylabel" {
      # "writes the private property \"ylabel\" to the plot object with the correct plotID"
      n183 = case shown="2" w447 {
        tunnel: w453 -> [_ _]
        tunnel: w452 -> [w454 w460]
        tunnel: [w454 w459] -> w451
        tunnel: w446 -> [_ w461]
        frame 0, Default {
          n184 = One Button Dialog(message="Not the right number of parameters!") -> ()  [unwired: 1 in, 1 out]
        }
        frame 2 {
          n185 = Index Array(array=w461) -> (element #1=w458:string, element #2=w457:string)  [unwired: 2 in]
          n186 = call "plot_set_labels.vi"("error in (no error)"=w460, "label"=w457, "axis"="ylabel", "plot name"=w458) -> ("error out"=w459:errorcluster)  [unwired: 7 in]
        }
      }
      n187 = global read "global variables.vi" "LogFileObj"() -> (w450:refnum<class "StatusLog.lvclass">)
      n188 = call-dynamic "add_log_entry.vi"("new entry"=w448, "log identifiers"="Script", "StatusLog in"=w450) -> ()  [unwired: 5 in, 2 out]
    }
    frame "plot_close" {
      # "closes the plot window by sending the plot command \"plot_close\""
      n189 = case shown="1" w462 {
        tunnel: w468 -> [w469 w477]
        tunnel: [w469 w475] -> w467
        tunnel: w463 -> [_ w474]
        frame 0, Default {
          n190 = One Button Dialog(message="Not the right number of parameters!") -> ()  [unwired: 1 in, 1 out]
        }
        frame 1 {
          # "plot name"
          n191 = call "PlotObjectArray_get_and_lock.vi"("error in (no error)"=w477) -> ("error out"=w473:errorcluster, "PlotObjects"=w479:refnum<class "Plots.lvclass">[])  [unwired: 9 in]
          n192 = call "find_PlotObject_by_Name.vi"("Plot Name/ID"=w474, "PlotObj Array in"=w479) -> ("index of Object in Array"=w480:i32, "found?"=w471:bool, "found PlotObj out"=w472:refnum<class "Plots.lvclass">)  [unwired: 6 in, 1 out]
          n193 = case shown="True" w471 {
            tunnel: w480 -> [_ w493]
            tunnel: w479 -> [w482 w491]
            tunnel: [w482 w490] -> w478
            tunnel: [w481 w489] -> w476
            tunnel: w473 -> [w481 w488]
            tunnel: w472 -> [_ w487]
            frame False {
            }
            frame True {
              n194 = To Variant(anything="") -> (Variant=w484:variant)
              n195 = Bundle("plot command"="plot_close", "Variant"=w484) -> (w485:T1)  [unwired: 1 in]
              n196 = call-dynamic "Write_plot-command.vi"("error in (no error)"=w488, "plot command"=w485, "Plots in"=w487) -> ("error out"=w489:errorcluster, "Plots out"=w492:refnum<class "Plots.lvclass">)  [unwired: 7 in]
              n197 = Replace Array Subset(array=w491, new element=w492, index=w493) -> (w490:refnum<class "Plots.lvclass">[])
            }
          }
          n198 = call "PlotObjectArray_write_and_unlock.vi"("error in (no error)"=w476, "PlotObjects"=w478) -> ("error out"=w475:errorcluster)  [unwired: 9 in]
        }
      }
      n199 = global read "global variables.vi" "LogFileObj"() -> (w466:refnum<class "StatusLog.lvclass">)
      n200 = call-dynamic "add_log_entry.vi"("new entry"=w464, "log identifiers"="Script", "StatusLog in"=w466) -> ()  [unwired: 5 in, 2 out]
    }
    frame "plot_find_single_peak" {
      # "plot_find_single_peak(plot_name;MFT_name;isotope_name(MFT);threshold)\ncommands the plot iven by plot_name to find a single peak in the plot data\nthe result of the peak centering is being updated in the magfield table --> it's important that the isotope_name is the same as in the MagFieldTable"
      n201 = case shown="4" w496 {
        tunnel: w499 -> [w503 w525]
        tunnel: w498 -> [_ _]
        tunnel: [w503 w517] -> w497
        tunnel: w494 -> [_ w513]
        tunnel: w495 -> [_ w509]
        frame 0, Default {
          n202 = One Button Dialog(message="Not the right number of parameters!") -> ()  [unwired: 1 in, 1 out]
        }
        frame 4 {
          # "it is not really necessary\nto also send the threshold\nwith the command\nsince the threshold is set in the\nprivate property if the plotObject\n\nthis is only useful to see the threshold\nin the plots status listbox"
          # "analysis session ID"
          # "update MagFieldTable"
          # "read peak centering result"
          # "isotope name"
          # "MFT name"
          # "- plot_name\n- MFT name\n- isotope_name (as given in MFT)\n- threshold"
          # "threshold"
          # "plot name"
          n203 = Index Array(array=w509) -> (element #1=w510:string, element #2=w508:string, element #3=w507:string, element #4=w506:string)  [unwired: 4 in]
          n204 = Fract/Exp String To Number(string=w506) -> (number=w505:dbl)  [unwired: 3 in, 1 out]
          n205 = call "PlotObjectArray_get_and_lock.vi"("error in (no error)"=w525) -> ("error out"=w523:errorcluster, "PlotObjects"=w527:refnum<class "Plots.lvclass">[])  [unwired: 9 in]
          n206 = call "find_PlotObject_by_Name.vi"("Plot Name/ID"=w510, "PlotObj Array in"=w527) -> ("index of Object in Array"=w528:i32, "found?"=w512:bool, "found PlotObj out"=w524:refnum<class "Plots.lvclass">)  [unwired: 6 in, 1 out]
          n207 = case shown="True" w512 {
            tunnel: w528 -> [_ w546]
            tunnel: w527 -> [w533 w545]
            tunnel: [w533 w544] -> w526
            tunnel: w524 -> [_ w543]
            tunnel: w523 -> [w532 w541]
            tunnel: w505 -> [_ w537]
            tunnel: [w532 w538] -> w522
            frame False {
            }
            frame True {
              n208 = call-dynamic "Write pc_threshold.vi"("error in (no error)"=w541, "pc_threshold"=w537, "Plots in"=w543) -> ("error out"=w540:errorcluster, "Plots out"=w542:refnum<class "Plots.lvclass">)  [unwired: 7 in]
              n209 = To Variant(anything=w537) -> (Variant=w536:variant)
              n210 = Bundle("format string"="plot_find_single_peak", "Variant"=w536) -> (w534:T2)  [unwired: 1 in]
              n211 = call-dynamic "Write_plot-command.vi"("error in (no error)"=w540, "plot command"=w534, "Plots in"=w542) -> ("error out"=w538:errorcluster, "Plots out"=w539:refnum<class "Plots.lvclass">)  [unwired: 7 in]
              n212 = Replace Array Subset(array=w545, new element=w539, index=w546) -> (w544:refnum<class "Plots.lvclass">[])
            }
          }
          n213 = call "PlotObjectArray_write_and_unlock.vi"("error in (no error)"=w522, "PlotObjects"=w526) -> ("error out"=w521:errorcluster)  [unwired: 9 in]
          n214 = call "Time Delay3"("error in (no error)"=w521) -> ("error out"=w520:errorcluster)  [unwired: 10 in]
          n215 = call "PlotObjectArray_get_and_lock.vi"("error in (no error)"=w520) -> ("error out"=w518:errorcluster, "PlotObjects"=w519:refnum<class "Plots.lvclass">[])  [unwired: 9 in]
          n216 = call "find_PlotObject_by_Name.vi"("Plot Name/ID"=w510, "PlotObj Array in"=w519) -> ("found?"=w511:bool, "found PlotObj out"=w515:refnum<class "Plots.lvclass">)  [unwired: 6 in, 2 out]
          n217 = call "PlotObjectArray_write_and_unlock.vi"("error in (no error)"=w518, "PlotObjects"=w519) -> ("error out"=w516:errorcluster)  [unwired: 9 in]
          n218 = case shown="True" w511 {
            tunnel: w515 -> [_ w531]
            tunnel: ["-99" ("result") w530] -> w514
            frame False {
            }
            frame True {
              n219 = call-dynamic "get_result_from_queue.vi"("Plots in"=w531) -> ("result"=w530:string)  [unwired: 8 in, 2 out]
            }
          }
          n220 = call "send_peakcenter_to_AnalysisObj.vi"("SessionID"=w513, "isotope name"=w507, "peak center value"=w514) -> ()  [unwired: 12 in, 1 out]
          n221 = case shown="\"true\", Default" w514 {
            selector: w514 -> [_ w549]
            tunnel: w508 -> [_ w552]
            tunnel: w507 -> [_ w551]
            tunnel: [w547 w550] -> w517
            tunnel: w516 -> [w547 w548]
            frame "-99" {
            }
            frame "true", Default {
              n222 = call "update_MagFieldTable.vi"("error in (no error)"=w548, "new magnet value"=w549, "isotope name"=w551, "MFT name"=w552) -> ("error out"=w550:errorcluster)  [unwired: 7 in]
            }
          }
        }
      }
      n223 = global read "global variables.vi" "LogFileObj"() -> (w502:refnum<class "StatusLog.lvclass">)
      n224 = call-dynamic "add_log_entry.vi"("new entry"=w500, "log identifiers"="Script", "StatusLog in"=w502) -> ()  [unwired: 5 in, 2 out]
    }
    frame "plot_find_double_peak" {
      # "plot_find_double_peak plot_name MFT_name isotope_name(MFT) threshold offset\n\ncommands the plot iven by plot_name to find a single peak in the plot data\nthe result of the peak centering is being updated in the magfield table --> it's important that the isotope_name is the same as in the MagFieldTable"
      n225 = global read "global variables.vi" "LogFileObj"() -> (w561:refnum<class "StatusLog.lvclass">)
      n226 = case shown="5" w555 {
        tunnel: w558 -> [w562 w586]
        tunnel: w557 -> [_ _]
        tunnel: [w562 w578] -> w556
        tunnel: w553 -> [_ w574]
        tunnel: w554 -> [_ w571]
        frame 0, Default {
          n227 = One Button Dialog(message="Not the right number of parameters!") -> ()  [unwired: 1 in, 1 out]
        }
        frame 5 {
          # "peaks offset"
          # "analysis session ID"
          # "update MagFieldTable"
          # "read peak centering result"
          # "isotope name"
          # "MFT name"
          # "- plot_name\n- MFT name\n- isotope_name (as given in MFT)\n- threshold\n- peaks offset"
          # "threshold"
          # "plot name"
          n228 = Index Array(array=w571) -> (element #1=w570:string, element #2=w569:string, element #3=w568:string, element #4=w567:string, element #5=w566:string)  [unwired: 5 in]
          n229 = Fract/Exp String To Number(string=w567) -> (number=w565:dbl)  [unwired: 3 in, 1 out]
          n230 = Fract/Exp String To Number(string=w566) -> (number=w564:dbl)  [unwired: 3 in, 1 out]
          n231 = call "PlotObjectArray_get_and_lock.vi"("error in (no error)"=w586) -> ("error out"=w584:errorcluster, "PlotObjects"=w588:refnum<class "Plots.lvclass">[])  [unwired: 9 in]
          n232 = call "find_PlotObject_by_Name.vi"("Plot Name/ID"=w570, "PlotObj Array in"=w588) -> ("index of Object in Array"=w589:i32, "found?"=w572:bool, "found PlotObj out"=w585:refnum<class "Plots.lvclass">)  [unwired: 6 in, 1 out]
          n233 = case shown="True" w572 {
            tunnel: w589 -> [_ w608]
            tunnel: w588 -> [w591 w607]
            tunnel: [w591 w606] -> w587
            tunnel: w585 -> [_ w605]
            tunnel: w584 -> [w590 w604]
            tunnel: w565 -> [_ w593]
            tunnel: [w590 w602] -> w583
            tunnel: w564 -> [_ w592]
            frame False {
            }
            frame True {
              n234 = call-dynamic "Write pc_threshold.vi"("error in (no error)"=w604, "pc_threshold"=w593, "Plots in"=w605) -> ("error out"=w600:errorcluster, "Plots out"=w601:refnum<class "Plots.lvclass">)  [unwired: 7 in]
              n235 = call-dynamic "Write pc_offset.vi"("error in (no error)"=w600, "pc_offset"=w592, "Plots in"=w601) -> ("error out"=w598:errorcluster, "Plots out"=w599:refnum<class "Plots.lvclass">)  [unwired: 7 in]
              n236 = Bundle(w593, w592) -> (w594:cluster{dbl, dbl})  [unwired: 1 in]
              n237 = To Variant(anything=w594) -> (Variant=w595:variant)
              n238 = Bundle("format string"="plot_find_double_peak", "Variant"=w595) -> (w596:T2)  [unwired: 1 in]
              n239 = call-dynamic "Write_plot-command.vi"("error in (no error)"=w598, "plot command"=w596, "Plots in"=w599) -> ("error out"=w602:errorcluster, "Plots out"=w603:refnum<class "Plots.lvclass">)  [unwired: 7 in]
              n240 = Replace Array Subset(array=w607, new element=w603, index=w608) -> (w606:refnum<class "Plots.lvclass">[])
            }
          }
          n241 = call "PlotObjectArray_write_and_unlock.vi"("error in (no error)"=w583, "PlotObjects"=w587) -> ("error out"=w582:errorcluster)  [unwired: 9 in]
          n242 = call "Time Delay5"("error in (no error)"=w582) -> ("error out"=w581:errorcluster)  [unwired: 10 in]
          n243 = call "PlotObjectArray_get_and_lock.vi"("error in (no error)"=w581) -> ("error out"=w579:errorcluster, "PlotObjects"=w580:refnum<class "Plots.lvclass">[])  [unwired: 9 in]
          n244 = call "find_PlotObject_by_Name.vi"("Plot Name/ID"=w570, "PlotObj Array in"=w580) -> ("found?"=w573:bool, "found PlotObj out"=w576:refnum<class "Plots.lvclass">)  [unwired: 6 in, 2 out]
          n245 = call "PlotObjectArray_write_and_unlock.vi"("error in (no error)"=w579, "PlotObjects"=w580) -> ("error out"=w577:errorcluster)  [unwired: 9 in]
          n246 = case shown="True" w573 {
            tunnel: w576 -> [_ w611]
            tunnel: ["-99" ("result") w610] -> w575
            frame False {
            }
            frame True {
              n247 = call-dynamic "get_result_from_queue.vi"("Plots in"=w611) -> ("result"=w610:string)  [unwired: 8 in, 2 out]
            }
          }
          n248 = case shown="\"true\", Default" w575 {
            selector: w575 -> [_ w614]
            tunnel: w569 -> [_ w617]
            tunnel: w568 -> [_ w616]
            tunnel: [w612 w615] -> w578
            tunnel: w577 -> [w612 w613]
            frame "-99" {
            }
            frame "true", Default {
              n249 = call "update_MagFieldTable.vi"("error in (no error)"=w613, "new magnet value"=w614, "isotope name"=w616, "MFT name"=w617) -> ("error out"=w615:errorcluster)  [unwired: 7 in]
            }
          }
          n250 = call "send_peakcenter_to_AnalysisObj.vi"("SessionID"=w574, "isotope name"=w568, "peak center value"=w575) -> ()  [unwired: 12 in, 1 out]
        }
      }
      n251 = call-dynamic "add_log_entry.vi"("new entry"=w559, "log identifiers"="Script", "StatusLog in"=w561) -> ()  [unwired: 5 in, 2 out]
    }
    frame "plot_fit_data" {
      # "plot_fit_data(plot_name;fityype[linear, 2nd, 3rd])\n\ncommands the plot to it the data by either linear, 2nd or 3rd order\nthe fit result is being saved in the AnalysisSession"
      n252 = global read "global variables.vi" "LogFileObj"() -> (w626:refnum<class "StatusLog.lvclass">)
      n253 = case shown="2" w621 {
        tunnel: w624 -> [w627 w647]
        tunnel: w623 -> [_ _]
        tunnel: [w627 w638] -> w622
        tunnel: w619 -> [_ w633]
        tunnel: w620 -> [_ w636]
        frame 0, Default {
          n254 = One Button Dialog(message="Not the right number of parameters!") -> ()  [unwired: 1 in, 1 out]
        }
        frame 2 {
          # "check if a session id excists\ni not don't send data o session object"
          # "fit type"
          # "it is not really necessary\nto also send the fit type\nwith the command\nsince the threshold is set in the\nprivate property if the plotObject\n\nthis is only useful to see the threshold\nin the plots status listbox"
          # "plot_name/isotope_name"
          # "read fit results"
          # "SessionID"
          # "- plot_name\n- fit type"
          # "plot name"
          n255 = Index Array(array=w636) -> (element #1=w635:string, element #2=w634:string)  [unwired: 2 in]
          n256 = call "PlotObjectArray_get_and_lock.vi"("error in (no error)"=w647) -> ("error out"=w645:errorcluster, "PlotObjects"=w649:refnum<class "Plots.lvclass">[])  [unwired: 9 in]
          n257 = call "find_PlotObject_by_Name.vi"("Plot Name/ID"=w635, "PlotObj Array in"=w649) -> ("index of Object in Array"=w650:i32, "found?"=w637:bool, "found PlotObj out"=w646:refnum<class "Plots.lvclass">)  [unwired: 6 in, 1 out]
          n258 = case shown="True" w637 {
            tunnel: w650 -> [_ w665]
            tunnel: w649 -> [w652 w664]
            tunnel: [w652 w663] -> w648
            tunnel: w646 -> [_ w662]
            tunnel: w645 -> [w651 w660]
            tunnel: [w651 w657] -> w644
            tunnel: w634 -> [_ w655]
            frame False {
            }
            frame True {
              n259 = To Variant(anything=w655) -> (Variant=w654:variant)
              n260 = call-dynamic "Write fit_type.vi"("error in (no error)"=w660, "fit_type"=w655, "Plots in"=w662) -> ("error out"=w659:errorcluster, "Plots out"=w661:refnum<class "Plots.lvclass">)  [unwired: 7 in]
              n261 = Bundle("format string"="plot_fit_data", "Variant"=w654) -> (w653:T2)  [unwired: 1 in]
              n262 = call-dynamic "Write_plot-command.vi"("error in (no error)"=w659, "plot command"=w653, "Plots in"=w661) -> ("error out"=w657:errorcluster, "Plots out"=w658:refnum<class "Plots.lvclass">)  [unwired: 7 in]
              n263 = Replace Array Subset(array=w664, new element=w658, index=w665) -> (w663:refnum<class "Plots.lvclass">[])
            }
          }
          n264 = call "PlotObjectArray_write_and_unlock.vi"("error in (no error)"=w644, "PlotObjects"=w648) -> ("error out"=w643:errorcluster)  [unwired: 9 in]
          n265 = call "Time Delay4"("error in (no error)"=w643) -> ("error out"=w642:errorcluster)  [unwired: 10 in]
          n266 = Empty String/Path?(string/path=w633) -> (empty?=w632:bool)
          n267 = Not(x=w632) -> (.not. x?=w630:bool)
          n268 = call "PlotObjectArray_get_and_lock.vi"("error in (no error)"=w642) -> ("error out"=w640:errorcluster, "PlotObjects"=w641:refnum<class "Plots.lvclass">[])  [unwired: 9 in]
          n269 = call "find_PlotObject_by_Name.vi"("Plot Name/ID"=w635, "PlotObj Array in"=w641) -> ("found?"=w631:bool, "found PlotObj out"=w639:refnum<class "Plots.lvclass">)  [unwired: 6 in, 2 out]
          n270 = And(x=w631, y=w630) -> (x .and. y?=w629:bool)
          n271 = call "PlotObjectArray_write_and_unlock.vi"("error in (no error)"=w640, "PlotObjects"=w641) -> ("error out"=w638:errorcluster)  [unwired: 9 in]
          n272 = case shown="True" w629 {
            tunnel: w639 -> [_ w674]
            tunnel: w635 -> [_ w669]
            tunnel: w633 -> [_ w667]
            tunnel: w634 -> [_ w666]
            frame False {
            }
            frame True {
              # "write extrapolation results into the\nAnalysisSession"
              n273 = call-dynamic "get_result_from_queue.vi"("Plots in"=w674) -> ("result"=w672:string)  [unwired: 8 in, 2 out]
              n274 = Scan From String(format string="intercept=%f, rmse=%f, delta-intercept=%f", input string=w672) -> (output 1=w671:dbl, output 2=w670:dbl, output 3=w668:dbl)  [unwired: 5 in, 3 out]
              n275 = call "send_ExptrapolResults_to_AnalysisObj.vi"("SessionID"=w667, "isotope name"=w669, "intercept"=w671, "RMSE"=w670, "delta-intercept"=w668, "fit type"=w666) -> ()  [unwired: 9 in, 1 out]
            }
          }
        }
      }
      n276 = call-dynamic "add_log_entry.vi"("new entry"=w625, "log identifiers"="Script", "StatusLog in"=w626) -> ()  [unwired: 5 in, 2 out]
    }
    frame "analysis_session_new" {
      # "If the analysis is triggered by a SampleList use the info given in the\nsample list, otherwise use the data from the command"
      # "update AnalysisSessionID string in the script\nwindow that called this command"
      # "The AnalysisSessionID is constructed\nfrom a timestamp at the moment of the\ncreation of the Session"
      # "analysis_session_new(ID,Name,Type)\n\nCreates a new analysis object\n\nThe object uses a internal SessionID to be indetified to other script processes.\n\nThe SessionID is created internally and is also saved to the Script that called\nthis command. In that wa avery script and it's subscripts knows what session to\nsave the data in.\nMultiple Scripts can run in parallel and have separate AnalysisSessions.\nTt saves AnalysisID, AnalysisName and AnalysisType\nthose infor will be used later to identify the \nif ID, name or type are not given a dialog appears"
      n277 = Array Size(array=w675) -> (size(s)=w678:i32)
      n278 = case shown="0, Default" w678 {
        tunnel: [w689 w700] -> w676
        tunnel: w677 -> [w689 _]
        tunnel: w675 -> [_ w700]
        frame 0, Default {
          # "it's not a sample list"
          n279 = Array To Spreadsheet String(array=w689, 3:"%s" ("format string")) -> (spreadsheet string=w692:string)  [unwired: 1 in]
          n280 = global read "global variables.vi" "LogFileObj"() -> (w695:refnum<class "StatusLog.lvclass">)
          n281 = Concatenate Strings("use Session Command info: " ("string"), w692) -> (w691:string)
          n282 = call-dynamic "add_log_entry.vi"("new entry"=w691, "log identifiers"="Script", "StatusLog in"=w695) -> ()  [unwired: 5 in, 2 out]
        }
        frame 1.. {
          # "it looks like the analysis comes from a sample list"
          n283 = Array To Spreadsheet String(array=w700, 3:"%s" ("format string")) -> (spreadsheet string=w698:string)  [unwired: 1 in]
          n284 = global read "global variables.vi" "LogFileObj"() -> (w702:refnum<class "StatusLog.lvclass">)
          n285 = Concatenate Strings("use SampleList info: " ("string"), w698) -> (w697:string)
          n286 = call-dynamic "add_log_entry.vi"("new entry"=w697, "log identifiers"="Script", "StatusLog in"=w702) -> ()  [unwired: 5 in, 2 out]
        }
      }
      n287 = global read "global variables.vi" "LogFileObj"() -> (w688:refnum<class "StatusLog.lvclass">)
      n288 = call-dynamic "add_log_entry.vi"("new entry"=w686, "log identifiers"="Script", "StatusLog in"=w688) -> ()  [unwired: 5 in, 2 out]
      n289 = Get Date/Time In Seconds() -> (seconds since 1Jan1904=w685:timestamp)
      n290 = Format Date/Time String(time format string (%c)="%Y%m%d%H%M%S", seconds (now)=w685) -> (date/time string=w681:string)  [unwired: 1 in]
      n291 = Build Array (concatenate)(w681, w676) -> (w680:string[])
      n292 = call "new_analysis.vi"("parameters"=w680) -> ()  [unwired: 11 in]
      n293 = property class="Str"(reference=w679, error in=w683, "Value"=w681) -> (error out=w682:errorcluster)  [unwired: 1 out]
    }
    frame "analysis_session_dump" {
      # "save the data to a file or database"
      # "analysis_session_dump\n\nAnalysisSessionID is stored in the Script that called this command.\nIn that way only this script and it's subscripts can have access to this paricular AnalysisSession.\n\nwrites the data stored in the AnalysisSession to a file or db etc etc"
      n294 = global read "global variables.vi" "LogFileObj"() -> (w703:refnum<class "StatusLog.lvclass">)
      n295 = call "AnalysisObjectArray_get_and_lock.vi"("error in (no error)"=w712) -> ("error out"=w714:errorcluster, "AnalysisObjects"=w713:refnum<class "Analysis.lvclass">[])  [unwired: 9 in]
      n296 = call-dynamic "add_log_entry.vi"("new entry"=w707, "log identifiers"="Script", "StatusLog in"=w703) -> ()  [unwired: 5 in, 2 out]
      n297 = call "find_AnalysisObject_by_SessionID.vi"("error in (no error)"=w714, "SessionID"=w705, "AnalysisObjects in"=w713) -> ("error out"=w704:errorcluster, "found AnalyisObject"=w709:refnum<class "Analysis.lvclass">, "AnalysisObjects out"=w710:refnum<class "Analysis.lvclass">[])  [unwired: 5 in, 1 out]
      n298 = call "Save_Data_To_File.vi"("error in (no error)"=w704, "Analysis in"=w709) -> ("error out"=w706:errorcluster)  [unwired: 8 in, 1 out]
      n299 = call "AnalysisObjectArray_write_and_unlock.vi"("error in (no error)"=w706, "AnalysisObjects"=w710) -> ("error out"=w711:errorcluster)  [unwired: 9 in]
    }
    frame "analysis_session_add_switch_counter" {
      # "analysis_session_add_switch_counter switch_name\n\nAnalysisSessionID is stored in the Script that called this command.\nIn that way only this script and it's subscripts can have access to this paricular AnalysisSession.\n\nstores the counter values of the switch in the CounterArray"
      n300 = case shown="1" w717 {
        tunnel: [w723 w729] -> w719
        tunnel: w716 -> [_ w728]
        tunnel: w718 -> [_ w727]
        tunnel: w715 -> [w723 w725]
        frame 0, Default {
          n301 = One Button Dialog(message="Not the right number of parameters!") -> ()  [unwired: 1 in, 1 out]
        }
        frame 1 {
          n302 = call "PrepLineObjectArray_get_and_lock_queue.vi"("error in (no error)"=w725) -> ("error out"=w734:errorcluster, "PrepLineObjects"=w736:refnum<class "PrepLineObject.lvclass">[])  [unwired: 9 in]
          n303 = call "find_PrepLineObject_by_Name.vi"("Name of Object"=w727, "PrepLineObjects in"=w736) -> ("found PrepLineObject"=w732:refnum<class "PrepLineObject.lvclass">, "PrepLineObjectsOut"=w735:refnum<class "PrepLineObject.lvclass">[], "found?"=w726:bool)  [unwired: 3 in, 3 out]
          n304 = call "PrepLineObjectArray_write_and_unlock_queue.vi"("error in (no error)"=w734, "PrepLineObjArray"=w735) -> ("error out"=w730:errorcluster)  [unwired: 9 in]
          n305 = case shown="True" w726 {
            tunnel: [u32 0 ("counter") w743] -> w733
            tunnel: w732 -> [_ w742]
            tunnel: ["counter??" ("name") w739] -> w731
            frame False {
            }
            frame True {
              n306 = call-dynamic "Read name.vi"("PrepLineObject in"=w742) -> ("error out"=w740:errorcluster, "name"=w739:string, "PrepLineObject out"=w741:refnum<class "PrepLineObject.lvclass">)  [unwired: 8 in]
              n307 = call-dynamic "Read_counter.vi"("error in (no error)"=w740, "PrepLineObject in"=w741) -> ("counter"=w743:u32)  [unwired: 7 in, 2 out]
            }
          }
          n308 = call "send_switch_counter_to_AnalysisObj.vi"("SessionID"=w728, "switch name"=w731, "counter value"=w733, "error in (no error)"=w730) -> ("error out"=w729:errorcluster)  [unwired: 11 in]
        }
      }
      n309 = global read "global variables.vi" "LogFileObj"() -> (w722:refnum<class "StatusLog.lvclass">)
      n310 = call-dynamic "add_log_entry.vi"("new entry"=w720, "log identifiers"="Script", "StatusLog in"=w722) -> ()  [unwired: 5 in, 2 out]
    }
    frame "analysis_session_add_standard_data" {
      # "analysis_session_add_standard_data(standard_name)\n\nAnalysisSessionID is stored in the Script that called this command.\nIn that way only this script and it's subscripts can have access to this paricular AnalysisSession.\n\nstores the data of the standard in the AnalysisSession"
      n311 = case shown="1" w746 {
        tunnel: [w752 w765] -> w748
        tunnel: w745 -> [_ w764]
        tunnel: w747 -> [_ w761]
        tunnel: w744 -> [w752 w754]
        frame 0, Default {
          n312 = One Button Dialog(message="Not the right number of parameters!") -> ()  [unwired: 1 in, 1 out]
        }
        frame 1 {
          n313 = call "StdObjectArray_get_and_lock.vi"("error in (no error)"=w754) -> ("error out"=w763:errorcluster, "StandardObjects"=w760:refnum<class "Standard.lvclass">[])  [unwired: 9 in]
          n314 = call "find_StdObject_by_Name.vi"("std_name"=w761, "StdObj Array in"=w760) -> ("found?"=w758:bool, "found StdObj out"=w757:refnum<class "Standard.lvclass">, "StdObj Array out"=w759:refnum<class "Standard.lvclass">[])  [unwired: 6 in, 1 out]
          n315 = call "StdObjectArray_write_and_unlock.vi"("error in (no error)"=w763, "StandardObjects"=w759) -> ("error out"=w762:errorcluster)  [unwired: 9 in]
          n316 = case shown="True" w758 {
            tunnel: w757 -> [_ w772]
            tunnel: [w768 w771] -> w766
            tunnel: [w768 w770] -> w756
            tunnel: [cluster{"isotope":string, "amount cc":dbl}[] [] ("Isotope Table") w769] -> w755
            frame False {
              w768 = "standard??" ("name")
            }
            frame True {
              n317 = call-dynamic "Read_name.vi"("Standard in"=w772) -> ("standard name"=w771:string)  [unwired: 8 in, 2 out]
              n318 = call-dynamic "Read-type.vi"("Standard in"=w772) -> ("type"=w770:string)  [unwired: 8 in, 2 out]
              n319 = call-dynamic "Read_Isotope-Table.vi"("Standard in"=w772) -> ("Isotope Table"=w769:cluster{"isotope":string, "amount cc":dbl}[])  [unwired: 8 in, 2 out]
            }
          }
          n320 = call "send_standard_to_AnalysisObj.vi"("SessionID"=w764, "standard_name"=w766, "standard_type"=w756, "Isotope Table"=w755, "error in (no error)"=w762) -> ("error out"=w765:errorcluster)  [unwired: 10 in]
        }
      }
      n321 = global read "global variables.vi" "LogFileObj"() -> (w751:refnum<class "StatusLog.lvclass">)
      n322 = call-dynamic "add_log_entry.vi"("new entry"=w749, "log identifiers"="Script", "StatusLog in"=w751) -> ()  [unwired: 5 in, 2 out]
    }
    frame "analysis_session_add_pipette_data" {
      # "analysis_session_add_pipette_data(pipette_name;number_of_shots)\n\nAnalysisSessionID is stored in the Script that called this command.\nIn that way only this script and it's subscripts can have access to this paricular AnalysisSession.\n\nstores the data of the pipette in the AnalysisSession"
      n323 = global read "global variables.vi" "LogFileObj"() -> (w780:refnum<class "StatusLog.lvclass">)
      n324 = case shown="2" w775 {
        tunnel: [w781 w799] -> w777
        tunnel: w774 -> [_ w798]
        tunnel: w776 -> [_ w789]
        tunnel: w773 -> [w781 w783]
        frame 0, Default {
          n325 = One Button Dialog(message="Not the right number of parameters!") -> ()  [unwired: 1 in, 1 out]
        }
        frame 2 {
          # "number of shots"
          n326 = call "PipObjectArray_get_and_lock.vi"("error in (no error)"=w783) -> ("error out"=w797:errorcluster, "PipObjects"=w795:refnum<class "Pipette.lvclass">[])  [unwired: 9 in]
          n327 = Match Pattern(string=w789, regular expression=";") -> (before substring=w788:string, after substring=w787:string)  [unwired: 1 in, 2 out]
          n328 = call "find_PipObject_by_Name.vi"("pipette_name"=w788, "PipObj Array in"=w795) -> ("found?"=w793:bool, "found PipObj out"=w792:refnum<class "Pipette.lvclass">, "PipObj Array out"=w794:refnum<class "Pipette.lvclass">[])  [unwired: 6 in, 1 out]
          n329 = call "PipObjectArray_write_and_unlock.vi"("error in (no error)"=w797, "PipObjects"=w794) -> ("error out"=w796:errorcluster)  [unwired: 9 in]
          n330 = case shown="True" w793 {
            tunnel: w792 -> [_ w802]
            tunnel: ["pipette??" ("name") w805] -> w800
            tunnel: [_ w804] -> w791
            tunnel: [_ w803] -> w790
            frame False {
            }
            frame True {
              n331 = call-dynamic "Read name.vi"("Pipette in"=w802) -> ("name"=w805:string)  [unwired: 8 in, 2 out]
              n332 = call-dynamic "Read dilution_factor.vi"("Pipette in"=w802) -> ("dilution_factor"=w804:dbl)  [unwired: 8 in, 2 out]
              n333 = call-dynamic "Read pipette counter.vi"("Pipette in"=w802) -> ("pipette counter"=w803:dbl)  [unwired: 8 in, 2 out]
            }
          }
          n334 = Decimal String To Number(string=w787, default (0L)=u32 0 ("default (0 I32)")) -> (number=w786:u32)  [unwired: 1 in, 1 out]
          n335 = call "send_pipette_to_AnalysisObj.vi"("SessionID"=w798, "pipette_name"=w800, "dilution factor"=w791, "pipette counter"=w790, "error in (no error)"=w796, "number of shots"=w786) -> ("error out"=w799:errorcluster)  [unwired: 9 in]
        }
      }
      n336 = call-dynamic "add_log_entry.vi"("new entry"=w778, "log identifiers"="Script", "StatusLog in"=w780) -> ()  [unwired: 5 in, 2 out]
    }
    frame "analysis_session_close" {
      # "analysis_session_close\n\nAnalysisSessionID is stored in the Script that called this command.\nIn that way only this script and it's subscripts can have access to this paricular AnalysisSession.\n\nremoves the AnalysisSessionObject from the global array"
      n337 = global read "global variables.vi" "LogFileObj"() -> (w808:refnum<class "StatusLog.lvclass">)
      n338 = call-dynamic "add_log_entry.vi"("new entry"=w806, "log identifiers"="Script", "StatusLog in"=w808) -> ()  [unwired: 5 in, 2 out]
      n339 = call "AnalysisObjectArray_get_and_lock.vi"() -> ("error out"=w816:errorcluster, "AnalysisObjects"=w815:refnum<class "Analysis.lvclass">[])  [unwired: 10 in]
      n340 = call "find_AnalysisObject_by_SessionID.vi"("error in (no error)"=w816, "SessionID"=w809, "AnalysisObjects in"=w815) -> ("error out"=w811:errorcluster, "index of found"=w812:i32, "AnalysisObjects out"=w814:refnum<class "Analysis.lvclass">[])  [unwired: 5 in, 1 out]
      n341 = Delete From Array(array=w814, length=1, index=w812) -> (array with subset deleted=w813:refnum<class "Analysis.lvclass">[])  [unwired: 1 out]
      n342 = call "AnalysisObjectArray_write_and_unlock.vi"("error in (no error)"=w811, "AnalysisObjects"=w813) -> ()  [unwired: 9 in, 1 out]
    }
    frame "set_time_zero" {
      # "set_time_zero(instrument)\n\nsets the time_zero to the instrument\nin all cases time zero is going to be saved as a private property\ndepending on the spectrometer time zero could also be written to the spectrometer"
      n343 = global read "global variables.vi" "LogFileObj"() -> (w823:refnum<class "StatusLog.lvclass">)
      n344 = call-dynamic "add_log_entry.vi"("new entry"=w821, "log identifiers"="Script", "StatusLog in"=w823) -> ()  [unwired: 5 in, 2 out]
      n345 = case shown="1" w817 {
        tunnel: w820 -> [_ w833]
        tunnel: w819 -> [w827 w829]
        tunnel: [w827 w828] -> w818
        frame 0, Default {
          w824 = "Not the right number of parameters!" ("message")
          n346 = global read "global variables.vi" "LogFileObj"() -> (w826:refnum<class "StatusLog.lvclass">)
          n347 = call-dynamic "add_log_entry.vi"("new entry"=w824, "log identifiers"="Script", "StatusLog in"=w826) -> ()  [unwired: 5 in, 2 out]
          n348 = One Button Dialog(message=w824) -> ()  [unwired: 1 in, 1 out]
        }
        frame 1 {
          n349 = call "InstrumentObjectArray_get_and_lock.vi"("error in (no error)"=w829) -> ("error out"=w831:errorcluster, "InstrumentsObjects"=w840:refnum<class "instrument.lvclass">[])  [unwired: 9 in]
          n350 = call "find_InstrumentObject_by_Name.vi"("Instrument Name"=w833, "InstrumentObjects"=w840) -> ("found?"=w832:bool, "index of found"=w839:i32, "found InstrObject out"=w836:refnum<class "instrument.lvclass">, "InstrumentObjects out"=w838:refnum<class "instrument.lvclass">[])  [unwired: 6 in]
          n351 = Get Date/Time In Seconds() -> (seconds since 1Jan1904=w835:timestamp)
          n352 = case shown="True" w832 {
            tunnel: w839 -> [_ w849]
            tunnel: w838 -> [w842 w848]
            tunnel: [w842 w847] -> w837
            tunnel: w836 -> [_ w846]
            tunnel: w835 -> [_ w845]
            tunnel: w831 -> [w841 w843]
            tunnel: [w841 w843] -> w830
            frame False {
            }
            frame True {
              n353 = call-dynamic "Write time zero.vi"("time zero"=w845, "instrument in"=w846) -> ("instrument out"=w844:refnum<class "instrument.lvclass">)  [unwired: 8 in, 1 out]
              n354 = Replace Array Subset(array=w848, new element=w844, index=w849) -> (w847:refnum<class "instrument.lvclass">[])
            }
          }
          n355 = call "InstrumentObjectArray_write_and_unlock.vi"("error in (no error)"=w830, "InstrumentObjects"=w837) -> ("error out"=w834:errorcluster)  [unwired: 9 in]
          n356 = call <vilib>:"Simple Error Handler.vi"("error in (no error)"=w834) -> ("error out"=w828:errorcluster)  [unwired: 4 in, 4 out]
        }
      }
    }
    frame "set_magnet" {
      # "set_magnet(instrument;value)\n\nset the magnet or controller of the instrument to the given value\nfor Qtegra value = MagnetDAC"
      n357 = global read "global variables.vi" "LogFileObj"() -> (w856:refnum<class "StatusLog.lvclass">)
      n358 = call-dynamic "add_log_entry.vi"("new entry"=w855, "log identifiers"="Script", "StatusLog in"=w856) -> ()  [unwired: 5 in, 2 out]
      n359 = case shown="2" w854 {
        tunnel: w857 -> [_ _]
        tunnel: w853 -> [w861 w866]
        tunnel: [w861 w865] -> w852
        tunnel: w851 -> [_ w864]
        frame 0, Default {
          w858 = "Not the right number of parameters!" ("message")
          n360 = global read "global variables.vi" "LogFileObj"() -> (w860:refnum<class "StatusLog.lvclass">)
          n361 = call-dynamic "add_log_entry.vi"("new entry"=w858, "log identifiers"="Script", "StatusLog in"=w860) -> ()  [unwired: 5 in, 2 out]
          n362 = One Button Dialog(message=w858) -> ()  [unwired: 1 in, 1 out]
        }
        frame 2 {
          n363 = Index Array(array=w864) -> (element #1=w863:string, element #2=w862:string)  [unwired: 2 in]
          n364 = call "InstrumentObjectArray_get_and_lock.vi"("error in (no error)"=w866) -> ("error out"=w873:errorcluster, "InstrumentsObjects"=w872:refnum<class "instrument.lvclass">[])  [unwired: 9 in]
          n365 = call "find_InstrumentObject_by_Name.vi"("Instrument Name"=w863, "InstrumentObjects"=w872) -> ("found?"=w867:bool, "found InstrObject out"=w869:refnum<class "instrument.lvclass">, "InstrumentObjects out"=w870:refnum<class "instrument.lvclass">[])  [unwired: 6 in, 1 out]
          n366 = call "isotope_to_value.vi"("MFT name"=w863, "magnet string in"=w862) -> ("magnet value out"=w868:dbl)  [unwired: 9 in]
          n367 = call "InstrumentObjectArray_write_and_unlock.vi"("error in (no error)"=w873, "InstrumentObjects"=w870) -> ("error out"=w871:errorcluster)  [unwired: 9 in]
          n368 = case shown="True" w867 {
            tunnel: w869 -> [_ w878]
            tunnel: w868 -> [_ w877]
            frame False {
              n369 = global read "global variables.vi" "LogFileObj"() -> (w876:refnum<class "StatusLog.lvclass">)
              n370 = call-dynamic "add_log_entry.vi"("new entry"="Instrument Object not found", "log identifiers"="Spectrometer", "StatusLog in"=w876) -> ()  [unwired: 5 in, 2 out]
            }
            frame True {
              n371 = call-dynamic "spec_set_magnet.vi"("value"=w877, "instrument in"=w878) -> ()  [unwired: 7 in, 3 out]
            }
          }
          n372 = call <vilib>:"Simple Error Handler.vi"("error in (no error)"=w871) -> ("error out"=w865:errorcluster)  [unwired: 4 in, 4 out]
        }
      }
    }
    frame "set_detector_deflection" {
      # "set_detector_deflection(instrument;detector_name;value)\n\nset the deflection voltage of the detector of the instrument"
      n373 = global read "global variables.vi" "LogFileObj"() -> (w885:refnum<class "StatusLog.lvclass">)
      n374 = call-dynamic "add_log_entry.vi"("new entry"=w884, "log identifiers"="Script", "StatusLog in"=w885) -> ()  [unwired: 5 in, 2 out]
      n375 = case shown="3" w883 {
        tunnel: w886 -> [_ _]
        tunnel: w882 -> [w890 w896]
        tunnel: [w890 w895] -> w881
        tunnel: w880 -> [_ w894]
        frame 0, Default {
          w887 = "Not the right number of parameters!" ("message")
          n376 = global read "global variables.vi" "LogFileObj"() -> (w889:refnum<class "StatusLog.lvclass">)
          n377 = call-dynamic "add_log_entry.vi"("new entry"=w887, "log identifiers"="Script", "StatusLog in"=w889) -> ()  [unwired: 5 in, 2 out]
          n378 = One Button Dialog(message=w887) -> ()  [unwired: 1 in, 1 out]
        }
        frame 3 {
          # "voltage"
          # "detector name"
          # "instrument"
          n379 = Index Array(array=w894) -> (element #1=w893:string, element #2=w892:string, element #3=w891:string)  [unwired: 3 in]
          n380 = call "InstrumentObjectArray_get_and_lock.vi"("error in (no error)"=w896) -> ("error out"=w902:errorcluster, "InstrumentsObjects"=w901:refnum<class "instrument.lvclass">[])  [unwired: 9 in]
          n381 = call "find_InstrumentObject_by_Name.vi"("Instrument Name"=w893, "InstrumentObjects"=w901) -> ("found?"=w897:bool, "found InstrObject out"=w898:refnum<class "instrument.lvclass">, "InstrumentObjects out"=w899:refnum<class "instrument.lvclass">[])  [unwired: 6 in, 1 out]
          n382 = call "InstrumentObjectArray_write_and_unlock.vi"("error in (no error)"=w902, "InstrumentObjects"=w899) -> ("error out"=w900:errorcluster)  [unwired: 9 in]
          n383 = case shown="True" w897 {
            tunnel: w898 -> [_ w909]
            tunnel: w892 -> [_ w908]
            tunnel: w891 -> [_ w907]
            frame False {
              n384 = global read "global variables.vi" "LogFileObj"() -> (w905:refnum<class "StatusLog.lvclass">)
              n385 = call-dynamic "add_log_entry.vi"("new entry"="Instrument Object not found", "log identifiers"="Spectrometer", "StatusLog in"=w905) -> ()  [unwired: 5 in, 2 out]
            }
            frame True {
              n386 = Decimal String To Number(string=w907) -> (number=w906:i32)  [unwired: 2 in, 1 out]
              n387 = call-dynamic "spec_set_deflection.vi"("deflection value"=w906, "detector name"=w908, "instrument in"=w909) -> ()  [unwired: 6 in, 3 out]
            }
          }
          n388 = call <vilib>:"Simple Error Handler.vi"("error in (no error)"=w900) -> ("error out"=w895:errorcluster)  [unwired: 4 in, 4 out]
        }
      }
    }
    frame "set_detector_supply" {
      # "set_detector_supply(instrument;detector_name;value)\n\nset the deflection voltage of the detector of the instrument"
      n389 = global read "global variables.vi" "LogFileObj"() -> (w916:refnum<class "StatusLog.lvclass">)
      n390 = call-dynamic "add_log_entry.vi"("new entry"=w915, "log identifiers"="Script", "StatusLog in"=w916) -> ()  [unwired: 5 in, 2 out]
      n391 = case shown="3" w914 {
        tunnel: w917 -> [_ _]
        tunnel: w913 -> [w921 w927]
        tunnel: [w921 w926] -> w912
        tunnel: w911 -> [_ w925]
        frame 0, Default {
          w918 = "Not the right number of parameters!" ("message")
          n392 = global read "global variables.vi" "LogFileObj"() -> (w920:refnum<class "StatusLog.lvclass">)
          n393 = call-dynamic "add_log_entry.vi"("new entry"=w918, "log identifiers"="Script", "StatusLog in"=w920) -> ()  [unwired: 5 in, 2 out]
          n394 = One Button Dialog(message=w918) -> ()  [unwired: 1 in, 1 out]
        }
        frame 3 {
          # "voltage"
          # "detector name"
          # "instrument"
          n395 = Index Array(array=w925) -> (element #1=w924:string, element #2=w923:string, element #3=w922:string)  [unwired: 3 in]
          n396 = call "InstrumentObjectArray_get_and_lock.vi"("error in (no error)"=w927) -> ("error out"=w933:errorcluster, "InstrumentsObjects"=w932:refnum<class "instrument.lvclass">[])  [unwired: 9 in]
          n397 = call "find_InstrumentObject_by_Name.vi"("Instrument Name"=w924, "InstrumentObjects"=w932) -> ("found?"=w928:bool, "found InstrObject out"=w929:refnum<class "instrument.lvclass">, "InstrumentObjects out"=w930:refnum<class "instrument.lvclass">[])  [unwired: 6 in, 1 out]
          n398 = call "InstrumentObjectArray_write_and_unlock.vi"("error in (no error)"=w933, "InstrumentObjects"=w930) -> ("error out"=w931:errorcluster)  [unwired: 9 in]
          n399 = case shown="True" w928 {
            tunnel: w929 -> [_ w940]
            tunnel: w923 -> [_ w939]
            tunnel: w922 -> [_ w938]
            frame False {
              n400 = global read "global variables.vi" "LogFileObj"() -> (w936:refnum<class "StatusLog.lvclass">)
              n401 = call-dynamic "add_log_entry.vi"("new entry"="Instrument Object not found", "log identifiers"="Spectrometer", "StatusLog in"=w936) -> ()  [unwired: 5 in, 2 out]
            }
            frame True {
              n402 = Decimal String To Number(string=w938) -> (number=w937:i32)  [unwired: 2 in, 1 out]
              n403 = call-dynamic "spec_set_supply.vi"("supply value"=w937, "detector name"=w939, "instrument in"=w940) -> ()  [unwired: 6 in, 3 out]
            }
          }
          n404 = call <vilib>:"Simple Error Handler.vi"("error in (no error)"=w931) -> ("error out"=w926:errorcluster)  [unwired: 4 in, 4 out]
        }
      }
    }
    frame "set_cupconfig" {
      # "set_cupconfig(instrument;cubconfig_name, subcupconfig_name)\n\nset the cup and subcup-configuration of the instrument to the given cup_name\nand subcupconfig_name\nthis mainly applies to Qtegra"
      n405 = global read "global variables.vi" "LogFileObj"() -> (w947:refnum<class "StatusLog.lvclass">)
      n406 = call-dynamic "add_log_entry.vi"("new entry"=w946, "log identifiers"="Script", "StatusLog in"=w947) -> ()  [unwired: 5 in, 2 out]
      n407 = case shown="3" w945 {
        tunnel: w948 -> [_ _]
        tunnel: w944 -> [w952 w958]
        tunnel: [w952 w957] -> w943
        tunnel: w942 -> [_ w956]
        frame 0, Default {
          w949 = "Not the right number of parameters!" ("message")
          n408 = global read "global variables.vi" "LogFileObj"() -> (w951:refnum<class "StatusLog.lvclass">)
          n409 = call-dynamic "add_log_entry.vi"("new entry"=w949, "log identifiers"="Script", "StatusLog in"=w951) -> ()  [unwired: 5 in, 2 out]
          n410 = One Button Dialog(message=w949) -> ()  [unwired: 1 in, 1 out]
        }
        frame 3 {
          # "subcupconfig"
          # "cupconfig"
          n411 = Index Array(array=w956) -> (element #1=w955:string, element #2=w954:string, element #3=w953:string)  [unwired: 3 in]
          n412 = call "InstrumentObjectArray_get_and_lock.vi"("error in (no error)"=w958) -> ("error out"=w964:errorcluster, "InstrumentsObjects"=w963:refnum<class "instrument.lvclass">[])  [unwired: 9 in]
          n413 = call "find_InstrumentObject_by_Name.vi"("Instrument Name"=w955, "InstrumentObjects"=w963) -> ("found?"=w959:bool, "found InstrObject out"=w960:refnum<class "instrument.lvclass">, "InstrumentObjects out"=w961:refnum<class "instrument.lvclass">[])  [unwired: 6 in, 1 out]
          n414 = call "InstrumentObjectArray_write_and_unlock.vi"("error in (no error)"=w964, "InstrumentObjects"=w961) -> ("error out"=w962:errorcluster)  [unwired: 9 in]
          n415 = case shown="True" w959 {
            tunnel: w960 -> [_ w980]
            tunnel: w954 -> [_ w981]
            tunnel: w953 -> [_ w972]
            frame False {
              n416 = global read "global variables.vi" "LogFileObj"() -> (w967:refnum<class "StatusLog.lvclass">)
              n417 = call-dynamic "add_log_entry.vi"("new entry"="Instrument Object not found", "log identifiers"="Spectrometer", "StatusLog in"=w967) -> ()  [unwired: 5 in, 2 out]
            }
            frame True {
              w976 = "Spectrometer" ("log identifiers")
              n418 = call <vilib>:"Trim Whitespace.vi"("string"=w981) -> ("trimmed string"=w969:string)  [unwired: 1 in]
              n419 = call <vilib>:"Trim Whitespace.vi"("string"=w972) -> ("trimmed string"=w968:string)  [unwired: 1 in]
              n420 = global read "global variables.vi" "LogFileObj"() -> (w979:refnum<class "StatusLog.lvclass">)
              n421 = call-dynamic "spec_get_cupconfiglist.vi"("instrument in"=w980) -> ("error out"=w974:errorcluster, "CupConfigList"=w978:string, "instrument out"=w975:refnum<class "instrument.lvclass">)  [unwired: 8 in]
              n422 = call-dynamic "add_log_entry.vi"("new entry"=w978, "log identifiers"=w976, "StatusLog in"=w979) -> ("StatusLog out"=w977:refnum<class "StatusLog.lvclass">)  [unwired: 5 in, 1 out]
              n423 = call-dynamic "spec_get_subcupconfig.vi"("error in (no error)"=w974, "CupConfig name"=w969, "instrument in"=w975) -> ("error out"=w970:errorcluster, "SubCupConfigList"=w973:string, "instrument out"=w971:refnum<class "instrument.lvclass">)  [unwired: 6 in]
              n424 = call-dynamic "add_log_entry.vi"("new entry"=w973, "log identifiers"=w976, "StatusLog in"=w977) -> ()  [unwired: 5 in, 2 out]
              n425 = call-dynamic "spec_set_cupconfig.vi"("error in (no error)"=w970, "supcub config name"=w968, "cup config name"=w969, "instrument in"=w971) -> ()  [unwired: 5 in, 3 out]
            }
          }
          n426 = call <vilib>:"Simple Error Handler.vi"("error in (no error)"=w962) -> ("error out"=w957:errorcluster)  [unwired: 4 in, 4 out]
        }
      }
    }
    frame "protect_detector" {
      # "protect_detector(qtegra,H1_CDD,1)"
      # "protect_detector(instrument;detector_name, flag)\n\nprotects the given detector of the given instrument"
      n427 = global read "global variables.vi" "LogFileObj"() -> (w988:refnum<class "StatusLog.lvclass">)
      n428 = call-dynamic "add_log_entry.vi"("new entry"=w987, "log identifiers"="Script", "StatusLog in"=w988) -> ()  [unwired: 5 in, 2 out]
      n429 = case shown="3" w986 {
        tunnel: w989 -> [_ _]
        tunnel: w985 -> [w993 w999]
        tunnel: [w993 w998] -> w984
        tunnel: w983 -> [_ w997]
        frame 0, Default {
          w990 = "Not the right number of parameters!" ("message")
          n430 = global read "global variables.vi" "LogFileObj"() -> (w992:refnum<class "StatusLog.lvclass">)
          n431 = call-dynamic "add_log_entry.vi"("new entry"=w990, "log identifiers"="Script", "StatusLog in"=w992) -> ()  [unwired: 5 in, 2 out]
          n432 = One Button Dialog(message=w990) -> ()  [unwired: 1 in, 1 out]
        }
        frame 3 {
          n433 = Index Array(array=w997) -> (element #1=w996:string, element #2=w995:string, element #3=w994:string)  [unwired: 3 in]
          n434 = call "InstrumentObjectArray_get_and_lock.vi"("error in (no error)"=w999) -> ("error out"=w1005:errorcluster, "InstrumentsObjects"=w1004:refnum<class "instrument.lvclass">[])  [unwired: 9 in]
          n435 = call "find_InstrumentObject_by_Name.vi"("Instrument Name"=w996, "InstrumentObjects"=w1004) -> ("found?"=w1000:bool, "found InstrObject out"=w1001:refnum<class "instrument.lvclass">, "InstrumentObjects out"=w1002:refnum<class "instrument.lvclass">[])  [unwired: 6 in, 1 out]
          n436 = call "InstrumentObjectArray_write_and_unlock.vi"("error in (no error)"=w1005, "InstrumentObjects"=w1002) -> ("error out"=w1003:errorcluster)  [unwired: 9 in]
          n437 = case shown="True" w1000 {
            tunnel: w1001 -> [_ w1012]
            tunnel: w995 -> [_ w1011]
            tunnel: w994 -> [_ w1010]
            frame False {
              n438 = global read "global variables.vi" "LogFileObj"() -> (w1008:refnum<class "StatusLog.lvclass">)
              n439 = call-dynamic "add_log_entry.vi"("new entry"="Instrument Object not found", "log identifiers"="Spectrometer", "StatusLog in"=w1008) -> ()  [unwired: 5 in, 2 out]
            }
            frame True {
              n440 = case shown="\"1\", Default" w1010 {
                tunnel: [TRUE FALSE] -> w1009
                frame "1", Default {
                }
                frame "0" {
                }
              }
              n441 = call-dynamic "spec_protect_detector.vi"("protect?"=w1009, "Detector Name"=w1011, "instrument in"=w1012) -> ()  [unwired: 6 in, 3 out]
            }
          }
          n442 = call <vilib>:"Simple Error Handler.vi"("error in (no error)"=w1003) -> ("error out"=w998:errorcluster)  [unwired: 4 in, 4 out]
        }
      }
    }
    frame "activate_ioncounter" {
      # "activate_ioncounter(instrument; flag)\n\nactivates or deactivates the ioncounter"
      n443 = global read "global variables.vi" "LogFileObj"() -> (w1021:refnum<class "StatusLog.lvclass">)
      n444 = call-dynamic "add_log_entry.vi"("new entry"=w1020, "log identifiers"="Script", "StatusLog in"=w1021) -> ()  [unwired: 5 in, 2 out]
      n445 = case shown="2" w1019 {
        tunnel: w1022 -> [_ _]
        tunnel: w1018 -> [w1026 w1031]
        tunnel: [w1026 w1030] -> w1017
        tunnel: w1016 -> [_ w1029]
        frame 0, Default {
          w1023 = "Not the right number of parameters!" ("message")
          n446 = global read "global variables.vi" "LogFileObj"() -> (w1025:refnum<class "StatusLog.lvclass">)
          n447 = call-dynamic "add_log_entry.vi"("new entry"=w1023, "log identifiers"="Script", "StatusLog in"=w1025) -> ()  [unwired: 5 in, 2 out]
          n448 = One Button Dialog(message=w1023) -> ()  [unwired: 1 in, 1 out]
        }
        frame 2 {
          n449 = Index Array(array=w1029) -> (element #1=w1028:string, element #2=w1027:string)  [unwired: 2 in]
          n450 = call "InstrumentObjectArray_get_and_lock.vi"("error in (no error)"=w1031) -> ("error out"=w1037:errorcluster, "InstrumentsObjects"=w1036:refnum<class "instrument.lvclass">[])  [unwired: 9 in]
          n451 = call "find_InstrumentObject_by_Name.vi"("Instrument Name"=w1028, "InstrumentObjects"=w1036) -> ("found?"=w1032:bool, "found InstrObject out"=w1033:refnum<class "instrument.lvclass">, "InstrumentObjects out"=w1034:refnum<class "instrument.lvclass">[])  [unwired: 6 in, 1 out]
          n452 = call "InstrumentObjectArray_write_and_unlock.vi"("error in (no error)"=w1037, "InstrumentObjects"=w1034) -> ("error out"=w1035:errorcluster)  [unwired: 9 in]
          n453 = case shown="True" w1032 {
            tunnel: w1033 -> [_ w1042]
            tunnel: w1027 -> [_ w1043]
            frame False {
              n454 = global read "global variables.vi" "LogFileObj"() -> (w1040:refnum<class "StatusLog.lvclass">)
              n455 = call-dynamic "add_log_entry.vi"("new entry"="Instrument Object not found", "log identifiers"="Spectrometer", "StatusLog in"=w1040) -> ()  [unwired: 5 in, 2 out]
            }
            frame True {
              n456 = case shown="\"0\"" w1043 {
                tunnel: [TRUE FALSE] -> w1041
                frame "1", Default {
                }
                frame "0" {
                }
              }
              n457 = call-dynamic "spec_set_ioncounter_state.vi"("state (on/off)"=w1041, "instrument in"=w1042) -> ()  [unwired: 7 in, 3 out]
            }
          }
          n458 = call <vilib>:"Simple Error Handler.vi"("error in (no error)"=w1035) -> ("error out"=w1030:errorcluster)  [unwired: 4 in, 4 out]
        }
      }
    }
    frame "signal_vs_magnet" {
      # "signal_vs_magnet(instrument;magnet_value;detector;integrtime;settling_time) -> plotname\n\nsets the magnet and integration times to specific values and returns the signal of the selected detector as well as the magnet value\nif plot is given plot the data.\nAnalysisSessionID is stored in the Script that called this command.\nIn that way only this script and it's subscripts can have access to this paricular AnalysisSession."
      n459 = global read "global variables.vi" "LogFileObj"() -> (w1056:refnum<class "StatusLog.lvclass">)
      n460 = case shown="5" w1050 {
        tunnel: w1053 -> [_ _]
        tunnel: [w1060 w1082] -> w1052
        tunnel: w1051 -> [_ w1081]
        tunnel: w1048 -> [_ w1075]
        tunnel: w1047 -> [w1060 w1074]
        tunnel: w1049 -> [_ w1072]
        tunnel: w1046 -> [_ w1063]
        frame 0, Default {
          w1057 = "Not the right number of parameters!" ("message")
          n461 = global read "global variables.vi" "LogFileObj"() -> (w1059:refnum<class "StatusLog.lvclass">)
          n462 = call-dynamic "add_log_entry.vi"("new entry"=w1057, "log identifiers"="Script", "StatusLog in"=w1059) -> ()  [unwired: 5 in, 2 out]
          n463 = One Button Dialog(message=w1057) -> ()  [unwired: 1 in, 1 out]
        }
        frame 5 {
          # "stop script if true (failed\nto read a datapoint)"
          # "settling time"
          # "send data\nin AnalysisSession\nin ScanArray"
          # "send the data\nto the plot"
          # "SessionID"
          # "instr\nmagnet\ndet\nintegr_time\nsettling_time"
          # "read value\ndetector value"
          # "set integration\ntime"
          # "set magnet"
          # "Integration_time +\n0.1 sec"
          n464 = Index Array(array=w1072) -> (element #1=w1071:string, element #2=w1070:string, element #3=w1069:string, element #4=w1068:string, element #5=w1066:string)  [unwired: 5 in]
          n465 = Fract/Exp String To Number(string=w1068) -> (number=w1067:dbl)  [unwired: 3 in, 1 out]
          n466 = Fract/Exp String To Number(string=w1066) -> (number=w1065:dbl)  [unwired: 3 in, 1 out]
          n467 = call "InstrumentObjectArray_get_and_lock.vi"("error in (no error)"=w1074) -> ("error out"=w1088:errorcluster, "InstrumentsObjects"=w1087:refnum<class "instrument.lvclass">[])  [unwired: 9 in]
          n468 = call "find_InstrumentObject_by_Name.vi"("Instrument Name"=w1071, "InstrumentObjects"=w1087) -> ("found InstrObject out"=w1084:refnum<class "instrument.lvclass">, "InstrumentObjects out"=w1086:refnum<class "instrument.lvclass">[])  [unwired: 6 in, 2 out]
          n469 = call "isotope_to_value.vi"("MFT name"=w1071, "magnet string in"=w1070) -> ("magnet value out"=w1080:dbl)  [unwired: 9 in]
          n470 = call "InstrumentObjectArray_write_and_unlock.vi"("error in (no error)"=w1088, "InstrumentObjects"=w1086) -> ("error out"=w1085:errorcluster)  [unwired: 9 in]
          n471 = call-dynamic "spec_set_magnet.vi"("value"=w1080, "instrument in"=w1084) -> ("error out"=w1078:errorcluster, "instrument out"=w1079:refnum<class "instrument.lvclass">)  [unwired: 7 in, 1 out]
          n472 = call <vilib>:"Simple Error Handler.vi"("error in (no error)"=w1085) -> ()  [unwired: 4 in, 5 out]
          n473 = call "Time Delay7"("error in (no error)"=w1078, "Delay Time (s)"=w1065) -> ("error out"=w1077:errorcluster)  [unwired: 9 in]
          n474 = call-dynamic "spec_set_integration_time.vi"("error in (no error)"=w1077, "integr time [s]"=w1067, "instrument in"=w1079) -> ("error out"=w1091:errorcluster, "instrument out"=w1089:refnum<class "instrument.lvclass">)  [unwired: 6 in, 1 out]
          n475 = Compound Arithmetic op=ADD(w1067, 0.2 ("y")) -> (w1083:dbl)
          n476 = call "Time Delay"("error in (no error)"=w1091, "Delay Time (s)"=w1083) -> ("error out"=w1090:errorcluster)  [unwired: 9 in]
          n477 = call-dynamic "spec_GetData.vi"("error in (no error)"=w1090, "Detector(s)"=w1069, "instrument in"=w1089) -> ("error out"=w1073:errorcluster, "failed?"=w1064:bool, "value(s)"=w1062:dbl[])  [unwired: 5 in, 1 out]
          n478 = Index Array(array=w1062) -> (element=w1061:dbl)  [unwired: 1 in]
          n479 = case shown="True" w1064 {
            selector: w1064 -> [_ w1092]
            tunnel: w1063 -> [_ w1094]
            frame False {
            }
            frame True {
              n480 = Not(x=w1092) -> (.not. x?=w1093:bool)
              n481 = To Variant(anything=w1093) -> (Variant=w1095:variant)
              n482 = property class="Bool"(reference=w1094, "Value"=w1095) -> ()  [unwired: 1 in, 2 out]
            }
          }
          n483 = call "send_data_to_plot.vi"("y-value"=w1061, "x-value"=w1080, "plotname"=w1081) -> ()  [unwired: 8 in, 1 out]
          n484 = call "send_scan_data_to_AnalysisObj.vi"("SessionID"=w1075, "plotname"=w1081, "magnet value in"=w1080, "value"=w1061, "error in (no error)"=w1073) -> ("error out"=w1082:errorcluster)  [unwired: 10 in]
        }
      }
      n485 = call-dynamic "add_log_entry.vi"("new entry"=w1054, "log identifiers"="Script", "StatusLog in"=w1056) -> ()  [unwired: 5 in, 2 out]
    }
    frame "OLD_signal_vs_time" {
      # "this command is not being used anymore"
      # "signal_vs_time(instrument;magnet_value;detector;integrtime;settling_time) -> plotname\n\nsets the magnet and integration times to specific values and returns the signal of the selected detector as well as the time elapsed since time zero\nif plot is given plot the data\nAnalysisSessionID is stored in the Script that called this command.\nIn that way only this script and it's subscripts can have access to this paricular AnalysisSession."
      n486 = global read "global variables.vi" "LogFileObj"() -> (w1106:refnum<class "StatusLog.lvclass">)
      n487 = case shown="5" w1100 {
        tunnel: w1103 -> [_ _]
        tunnel: w1102 -> [_ w1135]
        tunnel: w1098 -> [_ w1131]
        tunnel: w1097 -> [w1110 w1125]
        tunnel: [w1110 w1124] -> w1101
        tunnel: w1099 -> [_ w1123]
        tunnel: w1096 -> [_ w1113]
        frame 0, Default {
          w1107 = "Not the right number of parameters!" ("message")
          n488 = global read "global variables.vi" "LogFileObj"() -> (w1109:refnum<class "StatusLog.lvclass">)
          n489 = One Button Dialog(message=w1107) -> ()  [unwired: 1 in, 1 out]
          n490 = call-dynamic "add_log_entry.vi"("new entry"=w1107, "log identifiers"="Script", "StatusLog in"=w1109) -> ()  [unwired: 5 in, 2 out]
        }
        frame 5 {
          # "stop script if true (failed\nto read a datapoint)"
          # "set flag to 0 (good)"
          # "settling time"
          # "send data to AnalysisSession\nwill be saved later with\n\"analysis_session_dump\""
          # "Integration_time +\n0.5 sec"
          # "calculate time"
          # "Analysis SessionID"
          # "time"
          # "instr\nmagnet\ndet\nintegr_time\nsettling_time"
          # "get value\nfrom detector"
          # "set integration\ntime"
          # "set magnet"
          n491 = Index Array(array=w1123) -> (element #1=w1122:string, element #2=w1121:string, element #3=w1120:string, element #4=w1119:string, element #5=w1117:string)  [unwired: 5 in]
          n492 = Fract/Exp String To Number(string=w1119) -> (number=w1118:dbl)  [unwired: 3 in, 1 out]
          n493 = Fract/Exp String To Number(string=w1117) -> (number=w1116:dbl)  [unwired: 3 in, 1 out]
          n494 = call "InstrumentObjectArray_get_and_lock.vi"("error in (no error)"=w1125) -> ("error out"=w1142:errorcluster, "InstrumentsObjects"=w1141:refnum<class "instrument.lvclass">[])  [unwired: 9 in]
          n495 = call "isotope_to_value.vi"("MFT name"=w1122, "magnet string in"=w1121) -> ("magnet value out"=w1136:dbl)  [unwired: 9 in]
          n496 = call "find_InstrumentObject_by_Name.vi"("Instrument Name"=w1122, "InstrumentObjects"=w1141) -> ("found InstrObject out"=w1138:refnum<class "instrument.lvclass">, "InstrumentObjects out"=w1140:refnum<class "instrument.lvclass">[])  [unwired: 6 in, 2 out]
          n497 = call "InstrumentObjectArray_write_and_unlock.vi"("error in (no error)"=w1142, "InstrumentObjects"=w1140) -> ("error out"=w1139:errorcluster)  [unwired: 9 in]
          n498 = call-dynamic "spec_set_magnet.vi"("value"=w1136, "instrument in"=w1138) -> ("error out"=w1129:errorcluster, "instrument out"=w1130:refnum<class "instrument.lvclass">)  [unwired: 7 in, 1 out]
          n499 = call <vilib>:"Simple Error Handler.vi"("error in (no error)"=w1139) -> ()  [unwired: 4 in, 5 out]
          n500 = call-dynamic "spec_set_integration_time.vi"("error in (no error)"=w1129, "integr time [s]"=0.1, "instrument in"=w1130) -> ("error out"=w1127:errorcluster, "instrument out"=w1128:refnum<class "instrument.lvclass">)  [unwired: 6 in, 1 out]
          n501 = call "Time Delay6"("error in (no error)"=w1127, "Delay Time (s)"=w1116) -> ("error out"=w1133:errorcluster)  [unwired: 9 in]
          n502 = call-dynamic "spec_set_integration_time.vi"("error in (no error)"=w1133, "integr time [s]"=w1118, "instrument in"=w1128) -> ("error out"=w1147:errorcluster, "instrument out"=w1145:refnum<class "instrument.lvclass">)  [unwired: 6 in, 1 out]
          n503 = Compound Arithmetic op=ADD(w1118, 0.5 ("y")) -> (w1137:dbl)
          n504 = call "Time Delay2"("error in (no error)"=w1147, "Delay Time (s)"=w1137) -> ("error out"=w1146:errorcluster)  [unwired: 9 in]
          n505 = call-dynamic "spec_GetData.vi"("error in (no error)"=w1146, "Detector(s)"=w1120, "instrument in"=w1145) -> ("error out"=w1143:errorcluster, "failed?"=w1114:bool, "value(s)"=w1112:dbl[], "instrument out"=w1144:refnum<class "instrument.lvclass">)  [unwired: 5 in]
          n506 = stacked-sequence {
            tunnel: w1144 -> [w1152]
            tunnel: w1143 -> [w1153]
            tunnel: [w1154] -> w1134
            frame #0 {
              n507 = call-dynamic "Read time zero.vi"("error in (no error)"=w1153, "instrument in"=w1152) -> ("time zero"=w1155:timestamp)  [unwired: 7 in, 2 out]
              n508 = Get Date/Time In Seconds() -> (seconds since 1Jan1904=w1156:timestamp)
              n509 = Subtract(x=w1156, y=w1155) -> (x-y=w1154:dbl)
            }
          }
          n510 = case shown="True" w1114 {
            selector: w1114 -> [_ w1149]
            tunnel: w1113 -> [_ w1150]
            frame False {
            }
            frame True {
              n511 = Not(x=w1149) -> (.not. x?=w1148:bool)
              n512 = To Variant(anything=w1148) -> (Variant=w1151:variant)
              n513 = property class="Bool"(reference=w1150, "Value"=w1151) -> ()  [unwired: 1 in, 2 out]
            }
          }
          n514 = Index Array(array=w1112) -> (element=w1111:dbl)  [unwired: 1 in]
          n515 = call "send_data_to_plot.vi"("y-value"=w1111, "x-value"=w1134, "plotname"=w1135) -> ()  [unwired: 8 in, 1 out]
          n516 = call "send_analysis_data_to_AnalysisObj.vi"("SessionID"=w1131, "plotname"=w1135, "time in"=w1134, "value"=w1111, "flag in (0,1)"="0") -> ("error out"=w1124:errorcluster)  [unwired: 10 in]
        }
      }
      n517 = call-dynamic "add_log_entry.vi"("new entry"=w1104, "log identifiers"="Script", "StatusLog in"=w1106) -> ()  [unwired: 5 in, 2 out]
    }
    frame "signal_vs_time" {
      # "signal_vs_time(instrument;magnet_value;[detector1, detectror2,...];integrtime;settling_time) -> plotname1, plotname2,...\n\nsets the magnet and integration times to specific values and returns the signal of all of the given detectors as well as the time elapsed since time zero\nif plots are given plot the data: detector1->plotname1, detector2->plotname2\n\nAnalysisSessionID is stored in the Script that called this command.\nIn that way only this script and it's subscripts can have access to this paricular AnalysisSession."
      n518 = global read "global variables.vi" "LogFileObj"() -> (w1167:refnum<class "StatusLog.lvclass">)
      n519 = case shown="5" w1161 {
        tunnel: w1164 -> [_ _]
        tunnel: w1163 -> [_ w1176]
        tunnel: w1159 -> [_ w1193]
        tunnel: w1158 -> [w1171 w1187]
        tunnel: [w1171 w1186] -> w1162
        tunnel: w1160 -> [_ w1185]
        tunnel: w1157 -> [_ w1177]
        frame 0, Default {
          w1168 = "Not the right number of parameters!" ("message")
          n520 = global read "global variables.vi" "LogFileObj"() -> (w1170:refnum<class "StatusLog.lvclass">)
          n521 = One Button Dialog(message=w1168) -> ()  [unwired: 1 in, 1 out]
          n522 = call-dynamic "add_log_entry.vi"("new entry"=w1168, "log identifiers"="Script", "StatusLog in"=w1170) -> ()  [unwired: 5 in, 2 out]
        }
        frame 5 {
          # "detectors"
          # "plotname"
          # "stop script if true (failed\nto read a datapoint)"
          # "settling time"
          # "Integration_time +\n0.5 sec"
          # "calculate time"
          # "Analysis SessionID"
          # "time"
          # "instr\nmagnet \ndet's \nintegr_time\nsettling_time"
          # "get value from\neach detector"
          # "set integration\ntime"
          # "set magnet"
          n523 = Index Array(array=w1185) -> (element #1=w1184:string, element #2=w1183:string, element #3=w1172:string, element #4=w1182:string, element #5=w1180:string)  [unwired: 5 in]
          n524 = Fract/Exp String To Number(string=w1182) -> (number=w1181:dbl)  [unwired: 3 in, 1 out]
          n525 = Fract/Exp String To Number(string=w1180) -> (number=w1179:dbl)  [unwired: 3 in, 1 out]
          n526 = call "InstrumentObjectArray_get_and_lock.vi"("error in (no error)"=w1187) -> ("error out"=w1202:errorcluster, "InstrumentsObjects"=w1201:refnum<class "instrument.lvclass">[])  [unwired: 9 in]
          n527 = call "find_InstrumentObject_by_Name.vi"("Instrument Name"=w1184, "InstrumentObjects"=w1201) -> ("found InstrObject out"=w1198:refnum<class "instrument.lvclass">, "InstrumentObjects out"=w1200:refnum<class "instrument.lvclass">[])  [unwired: 6 in, 2 out]
          n528 = call "isotope_to_value.vi"("MFT name"=w1184, "magnet string in"=w1183) -> ("magnet value out"=w1196:dbl)  [unwired: 9 in]
          n529 = call "InstrumentObjectArray_write_and_unlock.vi"("error in (no error)"=w1202, "InstrumentObjects"=w1200) -> ("error out"=w1199:errorcluster)  [unwired: 9 in]
          n530 = call-dynamic "spec_set_magnet.vi"("value"=w1196, "instrument in"=w1198) -> ("error out"=w1191:errorcluster, "instrument out"=w1192:refnum<class "instrument.lvclass">)  [unwired: 7 in, 1 out]
          n531 = call <vilib>:"Simple Error Handler.vi"("error in (no error)"=w1199) -> ()  [unwired: 4 in, 5 out]
          n532 = call-dynamic "spec_set_integration_time.vi"("error in (no error)"=w1191, "integr time [s]"=0.1, "instrument in"=w1192) -> ("error out"=w1189:errorcluster, "instrument out"=w1190:refnum<class "instrument.lvclass">)  [unwired: 6 in, 1 out]
          n533 = call "Time Delay9"("error in (no error)"=w1189, "Delay Time (s)"=w1179) -> ("error out"=w1195:errorcluster)  [unwired: 9 in]
          n534 = call-dynamic "spec_set_integration_time.vi"("error in (no error)"=w1195, "integr time [s]"=w1181, "instrument in"=w1190) -> ("error out"=w1207:errorcluster, "instrument out"=w1205:refnum<class "instrument.lvclass">)  [unwired: 6 in, 1 out]
          n535 = Compound Arithmetic op=ADD(w1181, 0.5 ("y")) -> (w1197:dbl)
          n536 = call "Time Delay8"("error in (no error)"=w1207, "Delay Time (s)"=w1197) -> ("error out"=w1206:errorcluster)  [unwired: 9 in]
          n537 = call-dynamic "spec_GetData.vi"("error in (no error)"=w1206, "Detector(s)"=w1172, "instrument in"=w1205) -> ("error out"=w1203:errorcluster, "failed?"=w1178:bool, "value(s)"=w1173:dbl[], "instrument out"=w1204:refnum<class "instrument.lvclass">)  [unwired: 5 in]
          n538 = case shown="True" w1178 {
            selector: w1178 -> [_ w1215]
            tunnel: w1177 -> [_ w1216]
            frame False {
            }
            frame True {
              n539 = Not(x=w1215) -> (.not. x?=w1214:bool)
              n540 = To Variant(anything=w1214) -> (Variant=w1217:variant)
              n541 = property class="Bool"(reference=w1216, "Value"=w1217) -> ()  [unwired: 1 in, 2 out]
            }
          }
          n542 = stacked-sequence {
            tunnel: w1204 -> [w1218]
            tunnel: w1203 -> [w1219]
            tunnel: [w1220] -> w1174
            frame #0 {
              n543 = call-dynamic "Read time zero.vi"("error in (no error)"=w1219, "instrument in"=w1218) -> ("time zero"=w1221:timestamp)  [unwired: 7 in, 2 out]
              n544 = Get Date/Time In Seconds() -> (seconds since 1Jan1904=w1222:timestamp)
              n545 = Subtract(x=w1222, y=w1221) -> (x-y=w1220:dbl)
            }
          }
          n546 = call "convert_stringlist_to_array.vi"("string list"=w1176) -> ("array of strings"=w1175:string[])  [unwired: 4 in]
          n547 = for {
            tunnel: w1193 -> [w1213]
            tunnel: [w1212] -> w1186
            tunnel: w1175 -> [w1210] mode=indexing
            tunnel: w1174 -> [w1209]
            tunnel: w1173 -> [w1208] mode=indexing
            # "set flag to 0 (good)"
            n548 = call "send_data_to_plot.vi"("y-value"=w1208, "x-value"=w1209, "plotname"=w1210) -> ()  [unwired: 8 in, 1 out]
            n549 = call "send_analysis_data_to_AnalysisObj.vi"("SessionID"=w1213, "plotname"=w1210, "time in"=w1209, "value"=w1208, "flag in (0,1)"="0") -> ("error out"=w1212:errorcluster)  [unwired: 10 in]
          }
        }
      }
      n550 = call-dynamic "add_log_entry.vi"("new entry"=w1165, "log identifiers"="Script", "StatusLog in"=w1167) -> ()  [unwired: 5 in, 2 out]
    }
    frame "systemdevice_vs_time" {
      # "SessionID"
      # "plotname"
      # "systemdevice_vs_time(device_name) -> plotname\n\nread the value from a SystemDevice, return value and timestamp\nSystemDevice are pressure sensors and temperature readings"
      n551 = global read "global variables.vi" "LogFileObj"() -> (w1230:refnum<class "StatusLog.lvclass">)
      n552 = case shown="1" w1228 {
        tunnel: w1227 -> [_ _]
        tunnel: w1226 -> [_ w1237]
        tunnel: w1225 -> [_ w1256]
        tunnel: w1224 -> [_ _]
        tunnel: w1223 -> [_ w1236]
        frame 0, Default {
          w1232 = "Not the right number of parameters!" ("message")
          n553 = global read "global variables.vi" "LogFileObj"() -> (w1234:refnum<class "StatusLog.lvclass">)
          n554 = One Button Dialog(message=w1232) -> ()  [unwired: 1 in, 1 out]
          n555 = call-dynamic "add_log_entry.vi"("new entry"=w1232, "log identifiers"="Script", "StatusLog in"=w1234) -> ()  [unwired: 5 in, 2 out]
        }
        frame 1 {
          # "lock instrument so that no other process can perform writes\nor reads while this one is running"
          n556 = Index Array(array=w1256) -> (element=w1254:string)  [unwired: 1 in]
          n557 = call <vilib>:"Trim Whitespace.vi"("string"=w1254) -> ("trimmed string"=w1235:string)  [unwired: 1 in]
          n558 = call "PrepLineObjectArray_get_and_lock_queue.vi"() -> ("error out"=w1252:errorcluster, "PrepLineObjects"=w1255:refnum<class "PrepLineObject.lvclass">[])  [unwired: 10 in]
          n559 = call "find_PrepLineObject_by_Name.vi"("Name of Object"=w1235, "PrepLineObjects in"=w1255) -> ("found PrepLineObject"=w1245:refnum<class "PrepLineObject.lvclass">, "PrepLineObjectsOut"=w1253:refnum<class "PrepLineObject.lvclass">[])  [unwired: 3 in, 4 out]
          n560 = call "PrepLineObjectArray_write_and_unlock_queue.vi"("error in (no error)"=w1252, "PrepLineObjArray"=w1253) -> ()  [unwired: 9 in, 1 out]
          n561 = call-dynamic "Read_instrument-object.vi"("PrepLineObject in"=w1245) -> ("instrument.lvclass"=w1250:refnum<class "instrument.lvclass">)  [unwired: 8 in, 2 out]
          n562 = call-dynamic "Read_channel.vi"("PrepLineObject in"=w1245) -> ("channel"=w1244:u16, "PrepLineObject out"=w1242:refnum<class "PrepLineObject.lvclass">)  [unwired: 8 in, 1 out]
          n563 = call-dynamic "lock_semaphore.vi"("instrument in"=w1250) -> ("error out"=w1251:errorcluster, "instrument out"=w1246:refnum<class "instrument.lvclass">)  [unwired: 9 in]
          n564 = call-dynamic "get_value.vi"("error in (no error)"=w1251, "channel"=w1244, "instrument in"=w1246) -> ("error out"=w1248:errorcluster, "value"=w1243:string, "instrument out"=w1249:refnum<class "instrument.lvclass">)  [unwired: 6 in]
          n565 = call-dynamic "unlock_semaphore.vi"("error in (no error)"=w1248, "instrument in"=w1249) -> ()  [unwired: 8 in, 2 out]
          n566 = call-dynamic "convert_value.vi"("value in"=w1243, "PrepLineObject in"=w1242) -> ("converted value out"=w1241:string)  [unwired: 7 in, 2 out]
          n567 = Get Date/Time In Seconds() -> (seconds since 1Jan1904=w1247:timestamp)
          n568 = Fract/Exp String To Number(string=w1241) -> (number=w1239:dbl)  [unwired: 3 in, 1 out]
          n569 = To Double Precision Float(number=w1247) -> (double precision float=w1238:dbl)
          n570 = call "send_data_to_plot.vi"("y-value"=w1239, "x-value"=w1238, "plotname"=w1237) -> ()  [unwired: 8 in, 1 out]
          n571 = call "send_SystemDevice_data_to_AnalysisObj.vi"("SessionID"=w1236, "plotname"=w1235, "time in"=w1238, "value"=w1239, "flag in (0,1)"="0") -> ()  [unwired: 10 in, 1 out]
        }
      }
      n572 = call-dynamic "add_log_entry.vi"("new entry"=w1229, "log identifiers"="Script", "StatusLog in"=w1230) -> ()  [unwired: 5 in, 2 out]
    }
    frame "samplelist_proceed" {
      # "Sets the global flag (it's a flag object) \"SampleList_proceed\" to true and signals the SampleList Window t proceed to the next sample in the list"
      n573 = global read "global variables.vi" "LogFileObj"() -> (w1259:refnum<class "StatusLog.lvclass">)
      n574 = call-dynamic "add_log_entry.vi"("new entry"=w1257, "log identifiers"="Script", "StatusLog in"=w1259) -> ()  [unwired: 5 in, 2 out]
      n575 = call "FlagObjectArray_get_and_lock.vi"("error in (no error)"=w1261) -> ("error out"=w1263:errorcluster, "FlagObjects"=w1270:refnum<class "flag.lvclass">[])  [unwired: 9 in]
      n576 = call "find_FlagObject_by_Name.vi"("Flag Name"="SampleList_proceed", "FlagObj Array"=w1270) -> ("index of Object in Array"=w1265:i32, "found?"=w1264:bool, "found FlagObj out"=w1268:refnum<class "flag.lvclass">, "FlagObj Array out"=w1267:refnum<class "flag.lvclass">[])  [unwired: 6 in]
      n577 = case shown="True" w1264 {
        tunnel: w1268 -> [_ w1280]
        tunnel: w1267 -> [w1272 w1279]
        tunnel: [w1272 w1278] -> w1266
        tunnel: w1265 -> [_ w1277]
        tunnel: w1263 -> [w1271 w1275]
        tunnel: [w1271 w1274] -> w1262
        frame False {
        }
        frame True {
          n578 = call-dynamic "Write_flag-state.vi"("error in (no error)"=w1275, "flag state"=TRUE, "flag in"=w1280) -> ("error out"=w1274:errorcluster, "flag out"=w1276:refnum<class "flag.lvclass">)  [unwired: 7 in]
          n579 = Replace Array Subset(array=w1279, new element=w1276, index=w1277) -> (w1278:refnum<class "flag.lvclass">[])
        }
      }
      n580 = call "FlagObjectArray_write_and_unlock.vi"("error in (no error)"=w1262, "FlagObjects"=w1266) -> ("error out"=w1260:errorcluster)  [unwired: 9 in]
    }
  }
  "error out" <- w15
